vi "TH2829-20RunTest.vi"(0 "仪器通讯端口":refnum<visa-resource-name>, 6 "error in":errorcluster caption="错误输入（无错误）") -> (26 "error out":errorcluster caption="错误输出")   [LabVIEW 2018]
uses:
  Subvi/Global.vi
panel:
  out "数组 2":string[](array[string])
  out "数组":sgl[](array[numeric])
  out "子字符串":string
  out "read buffer":string
  out "Serial Settings:Number of Bytes at Serial Port":u32
  out "LED IrCompare Result":u8[][](array[numeric])
  out "LED IrResult":sgl[][](array[numeric]) format="%#_6f"
  out "总判断":u8
  out "Bls Result":sgl[][](array[numeric]) format="%#_6f"
  out "LED VfCompare Result":u8[][](array[numeric])
  out "LED VfResult":sgl[][](array[numeric]) format="%#_6f"
  out "PS Compare Result":u8[][](array[numeric])
  out "Polarity Result1":string[][](array[string])
  out "Rs Compare Result":u8[][](array[numeric])
  out "Z Compare Result":u8[][](array[numeric])
  out "Balance Compare Result":u8[][](array[numeric])
  out "LxQ Compare Result":u8[][](array[numeric])
  out "DCR Compare Result":u8[][](array[numeric])
  out "C Compare Result":u8[][](array[numeric])
  out "Lk Compare Result":u8[][](array[numeric])
  out "Lx Compare Result":u8[][](array[numeric])
  out "Turns Compare Result":u8[][](array[numeric])
  out "Polarity Result":u8[][](array[numeric])
  out "Zx Result":sgl[][](array[numeric]) format="%#_6f"
  out "ACR Result":sgl[][](array[numeric]) format="%#_6f"
  out "LxQ Result":sgl[][](array[numeric]) format="%#_6f"
  out "DCR Result":sgl[][](array[numeric]) format="%#_6f"
  out "Cx Result":sgl[][](array[numeric]) format="%#_6f"
  out "Lk Result":sgl[][](array[numeric]) format="%#_6f"
  out "Lx Result":sgl[][](array[numeric]) format="%#_6f"
  out "Turns Result":sgl[][](array[numeric]) format="%#_6f"
  out "Primary Sets":string
  out "head":string
  # "2304 0000 0000 0000 0000 0000 6041 E6C0 0B3D 0000 0000 F0A5 813C 0000 0000 0000 0000 0000 0000 0000 0000 0000 0000 0000 0000 0000 6041 3C18 E23C 0000 0000 CBA5 CD3B 0000 0000 0000 0000 0000 0000 0000 0000 0000 0000 0000 0000 0000 6041 D305 133D 0000 0000 5556 6A3C 0000 0000 0000 0000 0000 0000 0000 0000 0000 0000 0000 0000 0000 6041 A6B0 263D 0000 0000 2AAE 653C 0000 0000 0000 0000 0000 0000 0000 0000 0000 0000 0000 0000 0000 6041 072B 323D 0000 0000 A81B 993C 0000 0000 0000 0000 0000 0000 0000 0000 0000 0000 0000 0000 0000 6041 A94C 253D 0000 0000 D4A3 283C 0000 0000 0000 0000 0000 0000 0000 0000 0000 0000 0000 0000 0000 6041 849D 213D 0000 0000 39D1 7F3C 0000 0000 0000 0000 0000 0000 0000 0000 0000 0000 0000 0000 0000 6041 CA44 153D 0000 0000 3EC1 533C 0000 0000 0000 0000 0000 0000 0000 0000 0000 0000 0000 0000 0000 0000 0000 0000 0000 0000 0000 0000 0000 0000 0000 0000 0000 0000 0000 0000 0000 0000 0000 0000 0000 0000 0000 0000 0000 0000 0000 0000 0000 0000 0000 0000 0000 0000 0000 0000 0000 0000 0000 0000 0000 0000 0000 0000 0000 0000 0000 0000 0000 0000 0000 0000 0000 0000 0000 0000 0000 0000 0000 0000 0000 0000 0000 0000 0000 0000 0000 0000 0000 0000 0000 0000 0000 0000 0000 0000 0000 0000 0000 0000 0000 0000 0000 0000 0000 0000 0000 0000 0000 0000 0000 0000 0000 0000 0000 0000 0000 0000 0000 0000 0000 0000 0000 0000 0000 0000 0000 0000 0000 0000 0000 0000 0000 0000 0000 0000 0000 0000 0000 0000 0000 0000 0000 0000 0000 0000 0000 0000 0000 0000 0000 0000 0000 0000 0000 0000 0000 0000 0000 0000 0000 0000 0000 0000 0000 0000 0000 0000 0000 0000 0000 0000 0000 0000 0000 0000 0000 0000 0000 0000 0000 0000 0000 0000 0000 0000 0000 0000 0000 0000 0000 0000 0000 0000 0000 0000 0000 0000 0000 0000 0000 0000 0000 0000 0000 0000 0000 0000 0000 0000 0000 0000 0000 0000 0000 0000 0000 0000 0000 0000 0000 0000 0000 0000 0000 0000 0000 0000 0000 0000 0000 0000 0000 0000 0000 0000 0000 0000 0000 0000 0000 0000 0000 0000 0000 0000 0000 0000 0000 0000 0000 0000 0000 0000 0000 0000 0000 0000 0000 0000 0000 0000 0000 0000 0000 0000 0000 0000 0000 0000 0000 0000 0000 0000 0000 0000 0000 0000 0000 0000 0000 0000 0000 0000 0000 0000 0000 0000 0000 0000 0000 0000 0000 0000 0000 0000 0000 0000 0000 0000 0000 0000 0000 0000 0000 0000 0000 0000 0000 0000 0000 0000 0000 0000 0000 0000 0000 0000 0000 0000 0000 0000 0000 0000 0000 0000 0000 0000 0000 0000 0000 0000 0000 0000 0000 0000 0000 0000 0000 0000 0000 0000 0000 0000 0000 0000 0000 0000 0000 0000 0000 0000 0000 0000 0000 0000 0000 0000 0000 0000 0000 0000 0000 0000 0000 0000 0000 0000 0000 0000 0000 0000 0000 0000 0000 0000 0000 0000 0000 0000 0000 0000 0000 0000 0000 0000 0000 0000 0000 0000 0000 0000 0000 0000 0000 0000 0000 0000 0000 0000 0000 0000 0000 0000 0000 0000 0000 0000 0000 0000 0000 0000 0000 0000 0000 0000 0000 0000 0000 0000 0000 0000 0000 0000 0000 0000 0000 0000 0000 0000 0000 0000 0000 0000 0000 0000 0000 0000 0000 0000 0000 0000 0000 0000 0000 0000 0000 0000 0000 0000 0000 0000 0000 0000 0000 0000 0000 0000 0000 0000 0000 0000 0000 0000 0000 0000 0000 0000 0000 0000 0000 0000 0000 0000 0000 0000 0000 0000 0000 0000 0000 0000 0000 0000 0000 0000 0000 0000 0000 0000 0000 0000 0000 0000 0000 0000 0000 0000 0000 0000 0000 0000 0000 0000 0000 0000 0000 0000 0000 0000 0000 0000 0000 0000 0000 0000 0000 0000 0000 0000 0000 0000 0000 0000 0000 0000 0000 0000 0000 0000 0000 0000 0000 0000 0000 0000 0000 0000 0000 0000 0000 0000 0000 0000 0000 0000 0000 0000 0000 0000 0000 0000 0000 0000 0000 0000 0000 0000 0000 0000 0000 0000 0000 0000 0000 0000 0000 0000 0000 0000 0000 0000 0000 0000 0000 0000 0000 0000 0000 0000 0000 0000 0000 0000 0000 0000 0000 0000 0000 0000 0000 0000 0000 0000 0000 0000 0000 0000 0000 0000 0000 0000 0000 0000 0000 0000 0000 0000 0000 0000 0000 0000 0000 0000 0000 0000 0000 0000 0000 0000 0000 0000 0000 0000 0000 0000 0000 0000 0000 0000 0000 0000 0000 0000 0000 0000 0000 0000 0000 0000 0000 0000 0000 0000 0000 0000 0000 0000 0000 0000 0000 0000 0000 0000 0000 0000 0000 0000 0000 0000 F3AB 98BC 8E9F 1ABD 0000 0000 76B9 B1BD 0000 0000 0000 0000 0000 0000 0000 0000 0000 0000 0000 0000 75BB 8EBC 1715 01BD 0000 0000 76BC 77BD 0000 0000 0000 0000 0000 0000 0000 0000 0000 0000 0000 0000 A410 8FBC 4FD1 06BD 0000 0000 F5D1 79BD 0000 0000 0000 0000 0000 0000 0000 0000 0000 0000 0000 0000 DEEB A4BC 4F0C 15BD 0000 0000 485C 9CBD 0000 0000 0000 0000 0000 0000 0000 0000 0000 0000 0000 0000 06A7 86BC 0D51 1CBD 0000 0000 606A B1BD 0000 0000 0000 0000 0000 0000 0000 0000 0000 0000 0000 0000 209F A1BC 6393 02BD 0000 0000 2246 7BBD 0000 0000 0000 0000 0000 0000 0000 0000 0000 0000 0000 0000 AE0B 88BC 3FFC 07BD 0000 0000 BAB5 7FBD 0000 0000 0000 0000 0000 0000 0000 0000 0000 0000 0000 0000 459C 87BC C865 10BD 0000 0000 78DF 97BD 0000 0000 0000 0000 0000 0000 0000 0000 0000 0000 0000 0000 0000 0000 0000 0000 0000 0000 0000 0000 0000 0000 0000 0000 0000 0000 0000 0000 0000 0000 0000 0000 0000 0000 0000 0000 0000 0000 0000 0000 0000 0000 0000 0000 0000 0000 0000 0000 0000 0000 0000 0000 0000 0000 0000 0000 0000 0000 0000 0000 0000 0000 0000 0000 0000 0000 0000 0000 0000 0000 0000 0000 0000 0000 0000 0000 0000 0000 0000 0000 0000 0000 0000 0000 0000 0000 0000 0000 0000 0000 0000 0000 0000 0000 0000 0000 0000 0000 0000 0000 0000 0000 0000 0000 0000 0000 0000 0000 0000 0000 0000 0000 0000 0000 0000 0000 0000 0000 0000 0000 0000 0000 0000 0000 0000 0000 0000 0000 0000 0000 0000 0000 0000 0000 0000 0000 0000 0000 0000 0000 0000 0000 0000 0000 0000 0000 0000 0000 0000 0000 0000 0000 0000 0000 0000 0000 0000 0000 0000 0000 0000 0000 0000 0000 0000 0000 0000 0000 0000 0000 0000 0000 0000 0000 0000 0000 0000 0000 0000 0000 0000 0000 0000 0000 0000 0000 0000 0000 0000 0000 0000 0000 0000 0000 0000 0000 0000 0000 0000 0000 0000 0000 0000 0000 0000 0000 0000 0000 0000 0000 0000 0000 0000 0000 0000 0000 0000 0000 0000 0000 0000 0000 0000 0000 0000 0000 0000 0000 0000 0000 0000 0000 0000 0000 0000 0000 0000 0000 0000 0000 0000 0000 0000 0000 0000 0000 0000 0000 0000 0000 0000 0000 0000 0000 0000 0000 0000 0000 0000 0000 0000 0000 0000 0000 0000 0000 0000 0000 0000 0000 0000 0000 0000 0000 0000 0000 0000 0000 0000 0000 0000 0000 0000 0000 0000 0000 0000 0000 0000 0000 0000 0000 0000 0000 0000 0000 0000 0000 0000 0000 0000 0000 0000 0000 0000 0000 0000 0000 0000 0000 0000 0000 0000 0000 0000 0000 0000 0000 0000 0000 0000 0000 0000 0000 0000 0000 0000 0000 0000 0000 0000 0000 0000 0000 0000 0000 0000 0000 0000 0000 0000 0000 0000 0000 0000 0000 0000 0000 0000 0000 0000 0000 0000 0000 0000 0000 0000 0000 0000 0000 0000 0000 0000 0000 0000 0000 0000 0000 0000 0000 0000 0000 0000 0000 0000 0000 0000 0000 0000 0000 0000 0000 0000 0000 0000 0000 0000 0000 0000 0000 0000 0000 0000 0000 0000 0000 0000 0000 0000 0000 0000 0000 0000 0000 0000 0000 0000 0000 0000 0000 0000 0000 0000 0000 0000 0000 0000 0000 0000 0000 0000 0000 0000 0000 0000 0000 0000 0000 0000 0000 0000 0000 0000 0000 0000 0000 0000 0000 0000 0000 0000 0000 0000 0000 0000 0000 0000 0000 0000 0000 0000 0000 0000 0000 0000 0000 0000 0000 0000 0000 0000 0000 0000 0000 0000 0000 0000 0000 0000 0000 0000 0000 0000 0000 0000 0000 0000 0000 0000 0000 0000 0000 0000 0000 0000 0000 0000 0000 0000 0000 0000 0000 0000 0000 0000 0000 0000 0000 0000 0000 0000 0000 0000 0000 0000 0000 0000 0000 0000 0000 0000 0000 0000 0000 0000 0000 0000 0000 0000 0000 0000 0000 0000 0000 0000 0000 0000 0000 0000 0000 0000 0000 0000 0000 0000 0000 0000 0000 0000 0000 0000 0000 0000 0000 0000 0000 0000 0000 0000 0000 0000 0000 0000 0000 0000 0000 0000 0000 0000 0000 0000 0000 0000 0000 0000 0000 0000 0000 0000 0000 0000 0000 0000 0000 0000 0000 0000 0000 0000 0000 0000 0000 0000 0000 0000 0000 0000 0000 0000 0000 0000 0000 0000 0000 0000 0000 0000 0000 0000 0000 0000 0000 0000 0000 0000 0000 0000 0000 0000 0000 0000 0000 0000 0000 0000 0000 0000 0000 0000 0000 0000 0000 0000 0000 0000 0000 0000 0000 0000 0000 0000 0000 0000 0000 0000 0000 0000 0000 0000 0000 0000 0000 0000 0000 0000 0000 0000 0000 0000 0000 0000 0000 0000 0000 0000 0000 0000 0000 0000 0000 0000 0000 0000 0000 0000 0000 0000 0000 0000 0000 0000 0000 0000 0000 0000 0000 0000 0000 0000 0000 0000 0000 0000 0000 0000 0000 0000 0000 0000 0000 0000 0000 0000 0000 0000 0000 0000 0000 0000 0000 0000 0000 0000 0000 0000 0000 0000 0000 0000 0000 0000 0000 0000 0000 0000 0000 0000 0000 0000 0000 0000 0000 0000 0000 0000 0000 0000 0000 0000 0000 0000 0000 0000 0000 0000 0000 0000 0000 0000 0000 0000 0000 0000 0000 0000 0000 0000 0000 0000 0000 0000 0000 0000 0000 0000 0000 0000 0000 0000 0000 0000 0000 0000 0000 0000 0000 0000 0000 0000 0000 0000 0000 0000 0000 0000 0000 0000 0000 0000 0000 0000 0000 0000 0000 0000 0000 0000 0000 0000 0000 0000 0000 0000 0000 0000 0000 0000 0000 0000 0000 0000 0000 0000 0000 0000 0000 0000 0000 0000 0000 0000 0000 0000 0000 0000 0000 0000 0000 0000 0000 0000 0000 0000 0000 0000 0000 0000 0000 0000 0000 0000 0000 0000 0000 0000 0000 0000 0000 0000 0000 0000 0000 0000 0000 0000 0000 0000 0000 0000 0000 0000 0000 0000 0000 0000 0000 0000 0000 0000 0000 0000 0000 0000 0000 0000 0000 0000 0000 0000 0000 0000 0000 0000 0000 0000 0000 0000 0000 0000 0000 0000 0000 0000 0000 0000 0000 0000 0000 0000 0000 0000 0000 0000 0000 0000 0000 0000 0000 0000 0000 0000 0000 0000 0000 0000 0000 0000 0000 0000 0000 0000 0000 0000 0000 0000 0000 0000 0000 0000 0000 0000 0000 0000 0000 0000 0000 0000 0000 0000 0000 0000 0000 0000 0000 0000 0000 0000 0000 0000 0000 0000 0000 0000 0000 0000 0000 0000 0000 0000 0000 0000 0000 0000 0000 0000 0000 0000 0000 0000 0000 0000 0000 0000 0000 0000 0000 0000 0000 0000 0000 0000 0000 0000 0000 0000 0000 0000 0000 0000 0000 0000 0000 0000 0000 0000 0000 0000 0000 0000 0000 0000 0000 0000 0000 0000 0000 0000 0000 0000 0000 0000 0000 0000 0000 0000 0000 0000 0000 0000 0000 0000 0000 0000 0000 0000 0000 0000 0000 0000 0000 0000 0000 0000 0000 0000 0000 0000 0000 0000 0000 0000 0000 0000 0000 0000 0000 0000 0000 0000 0000 0000 0000 0000 0000 0000 0000 0000 0000 0000 0000 0000 0000 0000 0000 0000 0000 0000 0000 0000 0000 0000 0000 0000 0000 0000 0000 0000 0000 0000 0000 0000 0000 0000 0000 0000 0000 0000 0000 0000 0000 0000 0000 0000 0000 0000 0000 0000 0000 0000 0000 0000 0000 0000 0000 0000 0000 0000 0000 0000 0000 0000 0000 0000 0000 0000 0000 0000 0000 0000 0000 0000 0000 0000 0000 0000 0000 0000 0000 0000 0000 0000 0000 0000 0000 0000 0000 0000 0000 0000 0000 0000 0000 0000 0000 0000 0000 0000 0000 0000 0000 0000 0000 0000 0000 0000 0000 0000 0000 0000 0000 0000 0000 0000 0000 0000 0000 0000 0000 0000 0000 0000 0000 0000 0000 0000 0000 0000 0000 0000 0000 0000 0000 0000 0000 0000 0000 0000 0000 0000 0000 0000 0000 0000 0000 0000 0000 0000 0000 0000 0000 0000 0000 0000 0000 0000 0000 0000 0000 0000 0000 0000 0000 0000 0000 0000 0000 0000 0000 0000 0000 0000 0000 0000 0000 0000 0000 0000 0000 0000 0000 0000 0000 0000 0000 0000 0000 0000 0000 0000 0000 0000 0000 0000 0000 0000 0000 0000 0000 0000 0000 0000 0000 0000 0000 0000 0000 0000 0000 0000 0000 0000 0000 0000 0000 0000 0000 0000 0000 0000 0000 0000 0000 0000 0000 0000 0000 0000 0000 0000 0000 0000 0000 0000 0000 0000 0000 0000 0000 0000 0000 0000 0000 0000 0000 0000 0000 0000 0000 0000 0000 0000 0000 0000 0000 0000 0000 0000 0000 0000 0000 0000 0000 0000 0000 0000 0000 0000 0000 0000 0000 0000 0000 0000 0000 0000 0000 0000 0000 0000 0000 0000 0000 0000 0000 0000 0000 0000 0000 0000 0000 0000 0000 0000 0000 0000 0000 0000 0000 0000 0000 0000 0000 0000 0000 0000 0000 0000 0000 0000 0000 0000 0000 0000 0000 0000 0000 0000 0000 0000 0000 0000 0000 0000 0000 0000 0000 0000 0000 0000 0000 0000 0000 0000 0000 0000 0000 0000 0000 0000 0000 0000 0000 0000 0000 0000 0000 0000 0000 0000 0000 0000 0000 0000 0000 0000 0000 0000 0000 0000 0000 0000 0000 0000 0000 0000 0000 0000 0000 0000 0000 0000 0000 0000 0000 0000 0000 0000 0000 0000 0000 0000 0000 0000 0000 0000 0000 0000 0000 0000 0000 0000 0000 0000 0000 0000 0000 0000 0000 0000 0000 0000 0000 0000 0000 0000 0000 0000 0000 0000 0000 0000 0000 0000 0000 0000 0000 0000 0000 0000 0000 0000 0000 0000 0000 0000 0000 0000 0000 0000 0000 0000 0000 0000 0000 0000 0000 0000 0000 0000 0000 0000 0000 0000 0000 0000 0000 0000 0000 0000 0000 0000 0000 0000 0000 0000 0000 0000 0000 0000 0000 0000 0000 0000 0000 0000 0000 0000 0000 0000 0000 0000 0000 0000 0000 0000 0000 0000 0000 0000 0000 0000 0000 0000 0000 0000 0000 0000 0000 0000 0000 0000 0000 0000 0000 0000 0000 0000 0000 0000 0000 0000 0000 0000 0000 0000 0000 0000 0000 0000 0000 0000 0000 0000 0000 0000 0000 0000 0000 0000 0000 0000 0000 0000 0000 0000 0000 0000 0000 0000 0000 0000 0000 0000 0000 0000 0000 0000 0000 0000 0000 0000 0000 0000 0000 0000 0000 0000 0000 0000 0000 0000 0000 0000 0000 0000 0000 0000 0000 0000 0000 0000 0000 0000 0000 0000 0000 0000 0000 0000 0000 0000 0000 0000 0000 0000 0000 0000 0000 0000 0000 0000 0000 0000 0000 0000 0000 0000 0000 0000 0000 0000 0000 0000 0000 0000 0000 0000 0000 0000 0000 0000 0000 0000 0000 0000 0000 0000 0000 0000 0000 0000 0000 0000 0000 0000 0000 0000 0000 0000 0000 0000 0000 0000 0000 0000 0000 0000 0000 0000 0000 0000 0000 0000 0000 0000 0000 0000 0000 0000 0000 0000 0000 0000 0000 0000 0000 0000 0000 0000 0000 0000 0000 0000 0000 0000 0000 0000 0000 0000 0000 0000 0000 0000 0000 0000 0000 0000 0000 0000 0000 0000 0000 0000 0000 0000 0000 0000 0000 0000 0000 0000 0000 0000 0000 0000 0000 0000 0000 0000 0000 0000 0000 0000 0000 0000 0000 0000 0000 0000 0000 0000 0000 0000 0000 0000 0000 0000 0000 0000 0000 0000 0000 0000 0000 0000 0000 0000 0000 0000 0000 0000 0000 0000 0000 0000 0000 0000 0000 0000 0000 0000 0000 0000 0000 0000 0000 0000 0000 0000 0000 0000 0000 0000 0000 0000 0000 0000 0000 0000 0000 0000 0000 0000 0000 0000 0000 0000 0000 0000 0000 0000 0000 0000 0000 0000 0000 0000 0000 0000 0000 0000 0000 0000 0000 0000 0000 0000 0000 0000 0000 0000 0000 0000 0000 0000 0000 0000 0000 0000 0000 0000 0000 0000 0000 0000 0000 0000 0000 0000 0000 0000 0000 0000 0000 0000 0000 0000 0000 0000 0000 0000 0000 0000 0000 0000 0000 0000 0000 0000 0000 0000 0000 0000 0000 0000 0000 0000 0000 0000 0000 0000 0000 0000 0000 0000 0000 0000 0000 0000 0000 0000 0000 0000 0000 0000 0000 0000 0000 0000 0000 0000 0000 0000 0000 0000 0000 0000 0000 0000 0000 0000 0000 0000 0000 0000 0000 0000 0000 0000 0000 0000 0000 0000 0000 0000 0000 0000 0000 0000 0000 0000 0000 0000 0000 0000 0000 0000 0000 0000 0000 0000 0000 0000 0000 0000 0000 0000 0000 0000 0000 0000 0000 0000 0000 0000 0000 0000 0000 0000 0000 0000 0000 0000 0000 0000 0000 0000 0000 0000 0000 0000 0000 0000 0000 0000 0000 0000 0000 0000 0000 0000 0000 0000 0000 0000 0000 0000 0000 0000 0000 0000 0000 0000 0000 0000 0000 0000 0000 0000 0000 0000 0000 0000 0000 0000 0000 0000 0000 0000 0000 0000 0000 0000 0000 0000 0000 0000 0000 0000 0000 0000 0000 0000 0000 0000 0000 0000 0000 0000 0000 0000 0000 0000 0000 0000 0000 0000 0000 0000 0000 0000 0000 0000 0000 0000 0000 0000 0000 0000 0000 0000 0000 0000 0000 0000 0000 0000 0000 0000 0000 0000 0000 0000 0000 0000 0000 0000 0000 0000 0000 0000 0000 0000 0000 0000 0000 0000 0000 0000 0000 0000 0000 0000 0000 0000 0000 0000 0000 0000 0000 0000 0000 0000 0000 0000 0000 0000 0000 0000 0000 0000 0000 0000 0000 0000 0000 0000 0000 0000 0000 0000 0000 0000 0000 0000 0000 0000 0000 0000 0000 0000 0000 0000 0000 0000 0000 0000 0000 0000 0000 0000 0000 0000 0000 0000 0000 0000 0000 0000 0000 0000 0000 0000 0000 0000 0000 0000 0000 0000 0000 0000 0000 0000 0000 0000 0000 0000 0000 0000 0000 0000 0000 0000 0000 0000 0000 0000 0000 0000 0000 0000 0000 0000 0000 0000 0000 0000 0000 0000 0000 0000 0000 0000 0000 0000 0000 0000 0000 0000 0000 0000 0000 0000 0000 0000 0000 0000 0000 0000 0000 0000 0000 0000 0000 0000 0000 0000 0000 0000 0000 0000 0000 0000 0000 0000 0000 0000 0000 0000 0000 0000 0000 0000 0000 0000 0000 0000 0000 0000 0000 0000 0000 0000 0000 0000 0000 0000 0000 0000 0000 0000 0000 0000 0000 0000 0000 0000 0000 0000 0000 0000 0000 0000 0000 0000 0000 0000 0000 0000 0000 0000 0000 C79E 2E47 B30A 2148 6078 544C 3046 5A47 0000 0000 0000 0000 0000 0000 0000 0000 0000 0000 0000 0000 959E 2E47 2DF0 1048 6078 544C F446 5A47 0000 0000 0000 0000 0000 0000 0000 0000 0000 0000 0000 0000 FC9E 2E47 130B 2148 9CE8 3B4C 1547 5A47 0000 0000 0000 0000 0000 0000 0000 0000 0000 0000 0000 0000 7C9F 2E47 C3F0 1048 436B 744C 869F 2E47 0000 0000 0000 0000 0000 0000 0000 0000 0000 0000 0000 0000 ED90 2E47 9AE4 1048 7748 744C 0435 5A47 0000 0000 0000 0000 0000 0000 0000 0000 0000 0000 0000 0000 0991 2E47 82E4 1048 A648 744C 2435 5A47 0000 0000 0000 0000 0000 0000 0000 0000 0000 0000 0000 0000 A190 2E47 6FE4 1048 A648 744C DC90 2E47 0000 0000 0000 0000 0000 0000 0000 0000 0000 0000 0000 0000 8890 2E47 941D 3548 4A48 744C 2135 5A47 0000 0000 0000 0000 0000 0000 0000 0000 0000 0000 0000 0000 0000 0000 0000 0000 0000 0000 0000 0000 0000 0000 0000 0000 0000 0000 0000 0000 0000 0000 0000 0000 0000 0000 0000 0000 0000 0000 0000 0000 0000 0000 0000 0000 0000 0000 0000 0000 0000 0000 0000 0000 0000 0000 0000 0000 0000 0000 0000 0000 0000 0000 0000 0000 0000 0000 0000 0000 0000 0000 0000 0000 0000 0000 0000 0000 0000 0000 0000 0000 0000 0000 0000 0000 0000 0000 0000 0000 0000 0000 0000 0000 0000 0000 0000 0000 0000 0000 0000 0000 0000 0000 0000 0000 0000 0000 0000 0000 0000 0000 0000 0000 0000 0000 0000 0000 0000 0000 0000 0000 0000 0000 0000 0000 0000 0000 0000 0000 0000 0000 0000 0000 0000 0000 0000 0000 0000 0000 0000 0000 0000 0000 0000 0000 0000 0000 0000 0000 0000 0000 0000 0000 0000 0000 0000 0000 0000 0000 0000 0000 0000 0000 0000 0000 0000 0000 0000 0000 0000 0000 0000 0000 0000 0000 0000 0000 0000 0000 0000 0000 0000 0000 0000 0000 0000 0000 0000 0000 0000 0000 0000 0000 0000 0000 0000 0000 0000 0000 0000 0000 0000 0000 0000 0000 0000 0000 0000 0000 0000 0000 0000 0000 0000 0000 0000 0000 0000 0000 0000 0000 0000 0000 0000 0000 0000 0000 0000 0000 0000 0000 0000 0000 0000 0000 0000 0000 0000 0000 0000 0000 0000 0000 0000 0000 0000 0000 0000 0000 0000 0000 0000 0000 0000 0000 0000 0000 0000 0000 0000 0000 0000 0000 0000 0000 0000 0000 0000 0000 0000 0000 0000 0000 0000 0000 0000 0000 0000 0000 0000 0000 0000 0000 0000 0000 0000 0000 0000 0000 0000 0000 0000 0000 0000 0000 0000 0000 0000 0000 0000 0000 0000 0000 0000 0000 0000 0000 0000 0000 0000 0000 0000 0000 0000 0000 0000 0000 0000 0000 0000 0000 0000 0000 0000 0000 0000 0000 0000 0000 0000 0000 0000 0000 0000 0000 0000 0000 0000 0000 0000 0000 0000 0000 0000 0000 0000 0000 0000 0000 0000 0000 0000 0000 0000 0000 0000 0000 0000 0000 0000 0000 0000 0000 0000 0000 0000 0000 0000 0000 0000 0000 0000 0000 0000 0000 0000 0000 0000 0000 0000 0000 0000 0000 0000 0000 0000 0000 0000 0000 0000 0000 0000 0000 0000 0000 0000 0000 0000 0000 0000 0000 0000 0000 0000 0000 0000 0000 0000 0000 0000 0000 0000 0000 0000 0000 0000 0000 0000 0000 0000 0000 0000 0000 0000 0000 0000 0000 0000 0000 0000 0000 0000 0000 0000 0000 0000 0000 0000 0000 0000 0000 0000 0000 0000 0000 0000 0000 0000 0000 0000 0000 0000 0000 0000 0000 0000 0000 0000 0000 0000 0000 0000 0000 0000 0000 0000 0000 0000 0000 0000 0000 0000 0000 0000 0000 0000 0000 0000 0000 0000 0000 0000 0000 0000 0000 0000 0000 0000 0000 0000 0000 0000 0000 0000 0000 0000 0000 0000 0000 0000 0000 0000 0000 0000 0000 0000 0000 0000 0000 0000 0000 0000 0000 0000 0000 0000 0000 0000 0000 0000 0000 0000 0000 0000 0000 0000 0000 0000 0000 0000 0000 0000 0000 0000 0000 0000 0000 0000 0000 0000 0000 0000 0000 0000 0000 0000 0000 0000 0000 0000 0000 0000 0000 0000 0000 0000 0000 0000 0000 0000 0000 0000 0000 0000 0000 0000 0000 0000 0000 0000 0000 0000 0000 0000 0000 0000 0000 0000 0000 0000 0000 0000 0000 0000 0000 0000 0000 0000 0000 0000 0000 0000 0000 0000 0000 0000 0000 0000 0000 0000 0000 0000 0000 0000 0000 0000 0000 0000 0000 0000 0000 0000 0000 0000 0000 0000 0000 0000 0000 0000 0000 0000 0000 0000 0000 0000 0000 0000 0000 0000 0000 0000 0000 0000 0000 0000 0000 0000 0000 0000 0000 0000 0000 0000 0000 0000 0000 0000 0000 0000 0000 0000 0000 3B8C 48C3 E13C 88C2 0000 0000 E8AF C241 0000 0000 0000 0000 0000 0000 0000 0000 0000 0000 0000 0000 C165 2DC2 C9E0 C4C2 0000 0000 7FA3 1B42 0000 0000 0000 0000 0000 0000 0000 0000 0000 0000 0000 0000 832E 59C2 11B7 CB42 0000 0000 80F2 C541 0000 0000 0000 0000 0000 0000 0000 0000 0000 0000 0000 0000 CE1C F542 118C 09C3 0000 0000 D11B 0342 0000 0000 0000 0000 0000 0000 0000 0000 0000 0000 0000 0000 D29F 36C2 66F9 F8C2 0000 0000 1C9A A941 0000 0000 0000 0000 0000 0000 0000 0000 0000 0000 0000 0000 3882 DA41 CB53 EEC2 0000 0000 013E 1042 0000 0000 0000 0000 0000 0000 0000 0000 0000 0000 0000 0000 4C13 2A43 CF61 C542 0000 0000 318A BE41 0000 0000 0000 0000 0000 0000 0000 0000 0000 0000 0000 0000 1D63 0FC2 B6B2 B2C2 0000 0000 7420 0042 0000 0000 0000 0000 0000 0000 0000 0000 0000 0000 0000 0000 0000 0000 0000 0000 0000 0000 0000 0000 0000 0000 0000 0000 0000 0000 0000 0000 0000 0000 0000 0000 0000 0000 0000 0000 0000 0000 0000 0000 0000 0000 0000 0000 0000 0000 0000 0000 0000 0000 0000 0000 0000 0000 0000 0000 0000 0000 0000 0000 0000 0000 0000 0000 0000 0000 0000 0000 0000 0000 0000 0000 0000 0000 0000 0000 0000 0000 0000 0000 0000 0000 0000 0000 0000 0000 0000 0000 0000 0000 0000 0000 0000 0000 0000 0000 0000 0000 0000 0000 0000 0000 0000 0000 0000 0000 0000 0000 0000 0000 0000 0000 0000 0000 0000 0000 0000 0000 0000 0000 0000 0000 0000 0000 0000 0000 0000 0000 0000 0000 0000 0000 0000 0000 0000 0000 0000 0000 0000 0000 0000 0000 0000 0000 0000 0000 0000 0000 0000 0000 0000 0000 0000 0000 0000 0000 0000 0000 0000 0000 0000 0000 0000 0000 0000 0000 0000 0000 0000 0000 0000 0000 0000 0000 0000 0000 0000 0000 0000 0000 0000 0000 0000 0000 0000 0000 0000 0000 0000 0000 0000 0000 0000 0000 0000 0000 0000 0000 0000 0000 0000 0000 0000 0000 0000 0000 0000 0000 0000 0000 0000 0000 0000 0000 0000 0000 0000 0000 0000 0000 0000 0000 0000 0000 0000 0000 0000 0000 0000 0000 0000 0000 0000 0000 0000 0000 0000 0000 0000 0000 0000 0000 0000 0000 0000 0000 0000 0000 0000 0000 0000 0000 0000 0000 0000 0000 0000 0000 0000 0000 0000 0000 0000 0000 0000 0000 0000 0000 0000 0000 0000 0000 0000 0000 0000 0000 0000 0000 0000 0000 0000 0000 0000 0000 0000 0000 0000 0000 0000 0000 0000 0000 0000 0000 0000 0000 0000 0000 0000 0000 0000 0000 0000 0000 0000 0000 0000 0000 0000 0000 0000 0000 0000 0000 0000 0000 0000 0000 0000 0000 0000 0000 0000 0000 0000 0000 0000 0000 0000 0000 0000 0000 0000 0000 0000 0000 0000 0000 0000 0000 0000 0000 0000 0000 0000 0000 0000 0000 0000 0000 0000 0000 0000 0000 0000 0000 0000 0000 0000 0000 0000 0000 0000 0000 0000 0000 0000 0000 0000 0000 0000 0000 0000 0000 0000 0000 0000 0000 0000 0000 0000 0000 0000 0000 0000 0000 0000 0000 0000 0000 0000 0000 0000 0000 0000 0000 0000 0000 0000 0000 0000 0000 0000 0000 0000 0000 0000 0000 0000 0000 0000 0000 0000 0000 0000 0000 0000 0000 0000 0000 0000 0000 0000 0000 0000 0000 0000 0000 0000 0000 0000 0000 0000 0000 0000 0000 0000 0000 0000 0000 0000 0000 0000 0000 0000 0000 0000 0000 0000 0000 0000 0000 0000 0000 0000 0000 0000 0000 0000 0000 0000 0000 0000 0000 0000 0000 0000 0000 0000 0000 0000 0000 0000 0000 0000 0000 0000 0000 0000 0000 0000 0000 0000 0000 0000 0000 0000 0000 0000 0000 0000 0000 0000 0000 0000 0000 0000 0000 0000 0000 0000 0000 0000 0000 0000 0000 0000 0000 0000 0000 0000 0000 0000 0000 0000 0000 0000 0000 0000 0000 0000 0000 0000 0000 0000 0000 0000 0000 0000 0000 0000 0000 0000 0000 0000 0000 0000 0000 0000 0000 0000 0000 0000 0000 0000 0000 0000 0000 0000 0000 0000 0000 0000 0000 0000 0000 0000 0000 0000 0000 0000 0000 0000 0000 0000 0000 0000 0000 0000 0000 0000 0000 0000 0000 0000 0000 0000 0000 0000 0000 0000 0000 0000 0000 0000 0000 0000 0000 0000 0000 0000 0000 0000 0000 0000 0000 0000 0000 0000 0000 0000 0000 0000 0000 0000 0000 0000 0000 0000 0000 0000 0000 0000 0000 0000 0000 0000 0000 0000 0000 0000 0000 0000 0000 0000 0000 0000 0000 0000 0000 0000 0000 0000 0000 0000 0000 0000 0000 0000 0000 0000 0000 0000 0000 0000 0000 0000 0000 0000 0000 0000 0000 0000 0000 0000 0000 0000 0000 0000 0000 0000 0000 0000 0000 0000 0000 0000 0000 0000 0000 0000 0000 0000 0000 0000 0000 0000 0000 0000 0000 0000 0000 0000 0000 0000 0000 0000 0000 0000 0000 0000 0000 0000 0000 0000 0000 0000 0000 0000 0000 0000 0000 0000 0000 0000 0000 0000 0000 0000 0000 0000 0000 0000 0000 0000 0000 0000 0000 0000 0000 0000 0000 0000 0000 0000 0000 0000 0000 0000 0000 0000 0000 0000 0000 0000 0000 0000 0000 0000 0000 0000 0000 0000 0000 0000 0000 0000 0000 0000 0000 0000 0000 0000 0000 0000 0000 0000 0000 0000 0000 0000 0000 0000 0000 0000 0000 0000 0000 0000 0000 0000 0000 0000 0000 0000 0000 0000 0000 0000 0000 0000 0000 0000 0000 0000 0000 0000 0000 0000 0000 0000 0000 0000 0000 0000 0000 0000 0000 0000 0000 0000 0000 0000 0000 0000 0000 0000 0000 0000 0000 0000 0000 0000 0000 0000 0000 0000 0000 0000 0000 0000 0000 0000 0000 0000 0000 0000 0000 0000 0000 0000 0000 0000 0000 0000 0000 0000 0000 0000 0000 0000 0000 0000 0000 0000 0000 0000 0000 0000 0000 0000 0000 0000 0000 0000 0000 0000 0000 0000 0000 0000 0000 0000 0000 0000 0000 0000 0000 0000 0000 0000 0000 0000 0000 0000 0000 0000 0000 0000 0000 0000 0000 0000 0000 0000 0000 0000 0000 0000 0000 0000 0000 0000 0000 0000 0000 0000 0000 0000 0000 0000 0000 0000 0000 0000 0000 0000 0000 0000 0000 0000 0000 0000 0000 0000 0000 0000 0000 0000 0000 0000 0000 0000 0000 0000 0000 0000 0000 0000 0000 0000 0000 0000 0000 0000 0000 0000 0000 0000 0000 0000 0000 0000 0000 0000 0000 0000 0000 0000 0000 0000 0000 0000 0000 0000 0000 0000 0000 0000 0000 0000 0000 0000 0000 0000 0000 0000 0000 0000 0000 0000 0000 0000 0000 0000 0000 0000 0000 0000 0000 0000 0000 0000 0000 0000 0000 0000 0000 0000 0000 0000 0000 0000 0000 0000 0000 0000 0000 0000 0000 0000 0000 0000 0000 0000 0000 0000 0000 0000 0000 0000 0000 0000 0000 0000 0000 0000 0000 0000 0000 0000 0000 0000 0000 0000 0000 0000 0000 0000 0000 0000 0000 0000 0000 0000 0000 0000 0000 0000 0000 0000 0000 0000 0000 0000 0000 0000 0000 0000 0000 0000 0000 0000 0000 0000 0000 0000 0000 0000 0000 0000 0000 0000 0000 0000 0000 0000 0000 0000 0000 0000 0000 0000 0000 0000 0000 0000 0000 0000 0000 0000 0000 0000 0000 0000 0000 0000 0000 0000 0000 0000 0000 0000 0000 0000 0000 0000 0000 0000 0000 0000 0000 0000 0000 0000 0000 0000 0000 0000 0000 0000 0000 0000 0000 0000 0000 0000 0000 0000 0000 0000 0000 0000 0000 0000 0000 0000 0000 0000 0000 0000 0000 0000 0000 0000 0000 0000 0000 0000 0000 0000 0000 0000 0000 0000 0000 0000 0000 0000 0000 0000 0000 0000 0000 0000 0000 0000 0000 0000 0000 0000 0000 0000 0000 0000 0000 0000 0000 0000 0000 0000 0000 0000 0000 0000 0000 0000 0000 0000 0000 0000 0000 0000 0000 0000 0000 0000 0000 0000 0000 0000 0000 0000 0000 0000 0000 0000 0000 0000 0000 0000 0000 0000 0000 0000 0000 0000 0000 0000 0000 0000 0000 0000 0000 0000 0000 0000 0000 0000 0000 0000 0000 0000 0000 0000 0000 0000 0000 0000 0000 0000 0000 0000 0000 0000 0000 0000 0000 0000 0000 0000 0000 0000 0000 0000 0000 0000 0000 0000 0000 0000 0000 0000 0000 0000 0000 0000 0000 0000 0000 0000 0000 0000 0000 0000 0000 0000 0000 0000 0000 0000 0000 0000 0000 0000 0000 0000 0000 0000 0000 0000 0000 0000 0000 0000 0000 0000 0000 0000 0000 0000 0000 0000 0000 0000 0000 0000 0000 0000 0000 0000 0000 0000 0000 0000 0000 0000 0000 0000 0000 0000 0000 0000 0000 0000 0000 0000 0000 0000 0000 0000 0000 0000 0000 0000 0000 0000 0000 0000 0000 0000 0000 0000 0000 0000 0000 0000 0000 0000 0000 0000 0000 0000 0000 0000 0000 0000 0000 0000 0000 0000 0000 0000 0000 0000 0000 0000 0000 0000 0000 0000 0000 0000 0000 0000 0000 0000 0000 0000 0000 0000 0000 0000 0000 0000 0000 0000 0000 0000 0000 0000 0000 0000 0000 0000 0000 0000 0000 0000 0000 0000 0000 0000 0000 0000 0000 0000 0000 0000 0000 0000 0000 0000 0000 0000 0000 0000 0000 0000 0000 0000 0000 0000 0000 0000 0000 0000 0000 0000 0000 0000 0000 0000 0000 0000 0000 0000 0000 0000 0000 0000 0000 0000 0000 0000 0000 0000 0000 0000 0000 0000 0000 0000 0000 0000 0000 0000 0000 0000 0000 0000 0000 0000 0000 0000 0000 0000 0000 0000 0000 0000 0000 0000 0000 0000 0000 0000 0000 0000 0000 0000 0000 0000 0000 0000 0000 0000 0000 0000 0000 0000 0000 0000 0000 0000 0000 0000 0000 0000 0000 0000 0000 0000 0000 0000 0000 0000 0000 0000 0000 0000 0000 0000 0000 0000 0000 0000 0000 0000 0000 0000 0000 0000 0000 0000 0000 0000 0000 0000 0000 0000 0000 0000 0000 0000 0000 0000 0000 0000 0000 0000 0000 0000 0000 0000 0000 0000 0000 0000 0000 0000 0000 0000 0000 0000 0000 0000 0000 0000 0000 0000 0000 0000 0000 0000 0000 0000 0000 0000 0000 0000 0000 0000 0000 0000 0000 0000 0000 0000 0000 0000 0000 0000 0000 0000 0000 0000 0000 0000 0000 0000 0000 0000 0000 0000 0000 0000 0000 0000 0000 0000 0000 0000 0000 0000 0000 0000 0000 0000 0000 0000 0000 0000 0000 0000 0000 0000 0000 0000 0000 0000 0000 0000 0000 0000 0000 0000 0000 0000 0000 0000 0000 0000 0000 0000 0000 0000 0000 0000 0000 0000 0000 0000 0000 0000 0000 0000 0000 0000 0000 0000 0000 0000 0000 0000 0000 0000 0000 0000 0000 0000 0000 0000 0000 0000 0000 0000 0000 0000 0000 0000 0000 0000 0000 0000 0000 0000 0000 0000 0000 0000 0000 0000 0000 0000 0000 0000 0000 0000 0000 0000 0000 0000 0000 0000 0000 0000 0000 0000 0000 0000 0000 0000 0000 0000 0000 0000 0000 0000 0000 0000 0000 0000 0000 0000 0000 0000 0000 0000 0000 0000 0000 0000 0000 0000 0000 0000 0000 0000 0000 0000 0000 0000 0000 0000 0000 0000 0000 0000 0000 0000 0000 0000 0000 0000 0000 0000 0000 0000 0000 0000 0000 0000 0000 0000 0000 0000 0000 0000 0000 0000 0000 0000 0000 0000 0000 0000 0000 0000 0000 0000 0000 0000 0000 0000 0000 0000 0000 0000 0000 0000 0000 0000 0000 0000 0000 0000 0000 0000 0000 0000 0000 0000 0000 0000 0000 0000 0000 0000 0000 0000 0000 0000 0000 0000 0000 0000 0000 0000 0000 0000 0000 0000 0000 0000 0000 0000 0000 0000 0000 0000 0000 0000 0000 0000 0000 0000 0000 0000 0000 0000 0000 0000 0000 0000 0000 0000 0000 0000 0000 0000 0000 0000 0000 0000 0000 0000 0000 0000 0000 0000 0000 0000 0000 0000 0000 0000 0000 0000 0000 0000 0000 0000 0000 0000 0000 0000 0000 0000 0000 0000 0000 0000 0000 0000 0000 0000 0000 0000 0000 0000 0000 0000 0000 0000 0000 0000 0000 0000 0000 0000 0000 0000 0000 0000 0000 0000 0000 0000 0000 0000 0000 0000 0000 0000 0000 0000 0000 0000 0000 0000 0000 0000 0000 0000 0000 0000 0000 0000 0000 0000 0000 0000 0000 0000 0000 0000 0000 0000 0000 0000 0000 0000 0000 0000 0000 0000 0000 0000 0000 0000 0000 0000 0000 0000 0000 0000 0000 0000 0000 0000 0000 0000 0000 0000 0000 0000 0000 0000 0000 0000 0000 0000 0000 0000 0000 0000 0000 0000 0000 0000 0000 0000 0000 0000 0000 0000 0000 0000 0000 0000 0000 0000 0000 0000 0000 0000 0000 0000 0000 0000 0000 0000 0000 0000 0000 0000 0000 0000 0000 0000 0000 0000 0000 0000 0000 0000 0000 0000 0000 0000 0000 0000 0000 0000 0000 0000 0000 0000 0000 0000 0000 0000 0000 0000 0000 0000 0000 0000 0000 0000 0000 0000 0000 0000 0000 0000 0000 0000 0000 0000 0000 0000 0000 0000 0000 0000 0000 0000 0000 0000 0000 0000 0000 0000 0000 0000 0000 0000 0000 0000 0000 0000 0000 0000 0000 0000 0000 0000 0000 0000 0000 0000 0000 0000 0000 0000 0000 0000 0000 0000 0000 0000 0000 0000 0000 0000 0000 0000 0000 0000 0000 0000 0000 0000 0000 0000 0000 0000 0000 0000 0000 0000 0000 0000 0000 0000 0000 0000 0000 0000 0000 0000 0000 0000 0000 0000 0000 0000 0000 0000 0000 0000 0000 0000 0000 0000 0000 0000 0000 0000 0000 0000 0000 0000 0000 0000 0000 0000 0000 0000 0000 0000 0000 0000 0000 0000 0000 0000 0000 0000 0000 0000 0000 0000 0000 0000 0000 0000 0000 0000 0000 0000 0000 0000 0000 0000 0000 0000 0000 0000 0000 0000 0000 0000 0000 0000 0000 0000 0000 0000 0000 0000 0000 0000 0000 0000 0000 0000 0000 0000 0000 0000 0000 0000 0000 0000 0000 0000 0000 0000 0000 0000 0000 0000 0000 0000 0000 0000 0000 0000 0000 0000 0000 0000 0000 0000 0000 0000 0000 0000 0000 0000 0000 0000 0000 0000 0000 0000 0000 0000 0000 0000 0000 0000 0000 0000 0000 0000 0000 0000 0000 0000 0000 0000 0000 0000 0000 0000 0000 0000 0000 0000 0000 0000 0000 0000 0000 0000 0000 0000 0000 2B2D 202D 2020 2020 2020 2B2D 202D 2020 2020 2020 2B2D 202D 2020 2020 2020 2B2D 202D 2020 2020 2020 2B2D 202D 2020 2020 2020 2B2D 202D 2020 2020 2020 2B2D 202D 2020 2020 2020 2B2D 202D 2020 2020 2020 2020 2020 2020 2020 2020 2020 2020 2020 2020 2020 2020 2020 2020 2020 2020 2020 2020 2020 2020 2020 2020 2020 2020 2020 2020 2020 2020 2020 2020 2020 2020 2020 2020 2020 2020 2020 2020 2020 2020 2020 2020 2020 2020 2020 2020 2020 2020 2020 2020 2020 2020 2020 2020 2020 2020 2020 2020 2020 2020 2020 2020 2020 2020 2020 2020 2020 2020 2020 2020 2020 2020 2020 2020 2020 2020 2020 2020 2020 2020 2020 2020 2020 2020 2020 2020 2020 2020 2020 2020 2020 2020 2020 2020 2020 2020 2020 2020 2020 2020 2020 2020 2020 2020 2020 2020 2020 2020 2020 2020 2020 2020 2020 2020 2020 2020 2020 2020 2020 2020 2020 2020 2020 2020 2020 2020 2020 2020 2020 2020 2020 2020 2020 2020 2020 2020 2020 2020 2020 2020 2020 2020 2020 2020 2020 2020 2020 2020 2020 2020 2020 2020 2020 2020 2020 2020 2020 2020 2020 2020 2020 0002 0002 0000 0000 0000 0002 0002 0000 0000 0000 0002 0002 0000 0000 0000 0002 0002 0000 0000 0000 0002 0002 0000 0000 0000 0002 0002 0000 0000 0000 0002 0002 0000 0000 0000 0002 0002 0000 0000 0000 0000 0000 0000 0000 0000 0000 0000 0000 0000 0000 0000 0000 0000 0000 0000 0000 0000 0000 0000 0000 0000 0000 0000 0000 0000 0000 0000 0000 0000 0000 0000 0000 0000 0000 0000 0000 0000 0000 0000 0000 0000 0000 0000 0000 0000 0000 0000 0000 0000 0000 0000 0000 0000 0000 0000 0000 0000 0000 0000 0000 0000 0000 0000 0000 0000 0000 0000 0000 0000 0000 0000 0000 0000 0000 0000 0000 0000 0000 0000 0000 0000 0000 0000 0000 0000 0000 0000 0000 0000 0000 0000 0000 0000 0000 0000 0000 0000 0000 0000 0000 0000 0000 0000 0000 0000 0000 0000 0000 0000 0000 0000 0000 0000 0000 0000 0000 0000 0000 0000 0000 0000 0000 0000 0000 0000 0000 0000 0000 0000 0000 0000 0000 0000 0000 0000 0000 0000 0000 0000 0000 0000 0000 0000 0000 0000 0000 0000 0000 0000 0000 0000 0000 0000 0000 0000 0000 0000 0000 0000 0000 0202 0002 0000 0000 0000 0202 0002 0000 0000 0000 0202 0002 0000 0000 0000 0202 0002 0000 0000 0000 0202 0002 0000 0000 0000 0202 0002 0000 0000 0000 0202 0002 0000 0000 0000 0202 0002 0000 0000 0000 0000 0000 0000 0000 0000 0000 0000 0000 0000 0000 0000 0000 0000 0000 0000 0000 0000 0000 0000 0000 0000 0000 0000 0000 0000 0000 0000 0000 0000 0000 0000 0000 0000 0000 0000 0000 0000 0000 0000 0000 0000 0000 0000 0000 0000 0000 0000 0000 0000 0000 0000 0000 0000 0000 0000 0000 0000 0000 0000 0000 0000 0000 0000 0000 0000 0000 0000 0000 0000 0000 0000 0000 0000 0000 0000 0000 0000 0000 0000 0000 0000 0000 0000 0000 0000 0000 0000 0000 0000 0000 0000 0000 0000 0000 0000 0000 0000 0000 0000 0000 0000 0000 0000 0000 0000 0000 0000 0000 0000 0000 0000 0000 0000 0000 0000 0000 0000 0000 0000 0000 0000 0000 0000 0000 0000 0000 0000 0000 0000 0000 0000 0000 0000 0000 0000 0000 0000 0000 0000 0000 0000 0000 0000 0000 0000 0000 0000 0000 0000 0000 0000 0000 0000 0000 0000 0000 0000 0000 0000 0000 0000 0000 0000 0000 0000 0000 0000 0000 0000 0000 0000 0000 0000 0000 0000 0000 0000 0000 0000 0000 0000 0000 0000 0000 0000 0000 0000 0000 0000 0000 0000 0000 0000 0000 0000 0000 0000 0000 0000 0000 0000 0000 0000 0000 0000 0000 0000 0000 0000 0000 0000 0000 0000 0000 0000 0000 0000 0000 0000 0000 0000 0000 0000 0000 0000 0000 0000 0000 0000 0000 0000 0000 0000 0000 0000 0000 0000 0000 0000 0000 0000 0000 0000 0000 0000 0000 0000 0000 0000 0000 0000 0000 0000 0000 0000 0000 0000 0000 0000 0000 0000 0000 0000 0000 0000 0000 0000 0000 0000 0000 0000 0000 0000 0000 0000 0000 0000 0000 0000 0000 0000 0000 0000 0000 0000 0000 0000 0000 0000 0000 0000 0000 0000 0000 0000 0000 0000 0000 0000 0000 0000 0000 0000 0000 0000 0000 0000 0000 0000 0000 0000 0000 0000 0000 0000 0000 0000 0000 0000 0000 0000 0000 0000 0000 0000 0000 0000 0000 0000 0000 0000 0000 0000 0000 0000 0000 0000 0000 0000 0000 0000 0000 0000 0000 0000 0000 0000 0000 0000 0000 0000 0000 0000 0000 0000 0000 0000 0000 0000 0000 0000 0000 0000 0000 0000 0000 0000 0000 0000 0000 0000 0000 0000 0000 0000 0000 0000 0000 0000 0000 0000 0000 0000 0000 0000 0000 0000 0000 0000 0000 0000 0000 0000 0000 0000 0000 0000 0000 0000 0000 0000 0000 0000 0000 0000 0000 0000 0000 0000 0000 0000 0000 0000 0000 0000 0000 0000 0000 0000 0000 0000 0000 0000 0000 0000 0000 0000 0000 0000 0000 0000 0000 0000 0000 0000 0000 0000 0000 0000 0000 0000 0000 0000 0000 0000 0000 0000 0000 0000 0000 0000 0000 0000 0000 0000 0000 0000 0000 0000 0000 0000 0000 0000 0000 0000 0000 0000 0000 0000 0000 0000 0000 0000 0000 0000 0000 0000 0000 0000 0000 0000 0000 0000 0000 0000 0000 0000 0000 0000 0000 0000 0000 0000 0000 0000 0000 0000 0000 0000 0000 0000 0000 0000 0000 0000 0000 0000 0000 0000 0000 0000 0000 0000 0000 0000 0000 0000 0000 0000 0000 0000 0000 0000 0000 0000 0000 0000 0000 0000 0000 0000 0000 0000 0000 0000 0000 0000 0000 0000 0000 0000 0000 0000 0000 0000 0000 0000 0000 0000 0000 0000 0000 0000 0000 0000 0000 0000 0000 0000 0000 0303 0303 0000 0000 0000 0303 0303 0000 0000 0000 0303 0303 0000 0000 0000 0303 0303 0000 0000 0000 0303 0303 0000 0000 0000 0303 0303 0000 0000 0000 0303 0303 0000 0000 0000 0303 0303 0000 0000 0000 0000 0000 0000 0000 0000 0000 0000 0000 0000 0000 0000 0000 0000 0000 0000 0000 0000 0000 0000 0000 0000 0000 0000 0000 0000 0000 0000 0000 0000 0000 0000 0000 0000 0000 0000 0000 0000 0000 0000 0000 0000 0000 0000 0000 0000 0000 0000 0000 0000 0000 0000 0000 0000 0000 0000 0000 0000 0000 0000 0000 0000 0000 0000 0000 0000 0000 0000 0000 0000 0000 0000 0000 0000 0000 0000 0000 0000 0000 0000 0000 0000 0000 0000 0000 0000 0000 0000 0000 0000 0000 0000 0000 0000 0000 0000 0000 0000 0000 0000 0000 0000 0000 0000 0000 0000 0000 0000 0000 0000 0000 0000 0000 0000 0000 0000 0000 0000 0000 0000 0000 0000 0000 0000 0000 0000 0000 0000 0000 0000 0000 0000 0000 0000 0000 0000 0000 0000 0000 0000 0000 0000 0000 0000 0000 0000 0000 0000 0000 0000 0000 0000 0000 0000 0000 0000 0000 0000 0000 0000 0000 0000 0000 0000 0000 0000 0000 0000 0000 0000 0000 0000 0000 0000 0000 0000 0000 0000 0000 0000 0000 0000 0000 0000 0000 0000 0000 0000 0000 0000 0000 0000 0000 0000 0000 0000 0000 0000 0000 0000 0000 0000 0000 0000 0000 0000 0000 0000 0000 0000 0000 0000 0000 0000 0000 0000 0000 0000 0000 0000 0000 0000 0000 0000 0000 0000 0000 0000 0000 0000 0000 0000 0000 0000 0000 0000 0000 0000 0000 0000 0000 0000 0000 0000 0000 0000 0000 0000 0000 0000 0000 0000 0000 0000 0000 0000 0000 0000 0000 0000 0000 0000 0000 0000 0000 0000 0000 0000 0000 0000 0000 0000 0000 0000 0000 0000 0000 0000 0000 0000 0000 0000 0000 0000 0000 0000 0000 0000 0000 0000 0000 0000 0000 0000 0000 0000 0000 0000 0000 0000 0000 0000 0000 0000 0000 0000 0000 0000 0000 0000 0000 0000 0000 0000 0000 0000 0000 0000 0000 0000 0000 0000 0000 0000 0000 0000 0000 0000 0000 0000 0000 0000 0000 0000 0000 0000 0000 0000 0000 0000 0000 0000 0000 0000 0000 0000 0000 0000 0000 0000 0000 0000 0000 0000 0000 0000 0000 0000 0000 0000 0000 0000 0000 0000 0000 0000 0000 0000 0000 0000 0000 0000 0000 0000 0000 0000 0000 0000 0000 0000 0000 0000 0000 0000 0000 0000 0000 0000 0000 0000 0000 0000 0000 0000 0000 0000 0000 0000 0000 0000 0000 0000 0000 0000 0000 0000 0000 0000 0000 0000 0000 0000 0000 0000 0000 0000 0000 0000 0000 0000 0000 0000 0000 0000 0000 0000 0000 0000 0000 0000 0000 0000 0000 0000 0000 0000 0000 0000 0000 0000 0000 0000 0000 0000 0000 0000 0000 0000 0000 0000 0000 0000 0000 0000 0000 0000 0000 0000 0000 0000 0000 0000 0000 0000 0000 0000 0000 0000 0000 0000 0000 0000 0000 0000 0000 0000 0000 0000 0000 0000 0000 0000 0000 0000 0000 0000 0000 0000 0000 0000 0000 0000 0000 0000 0000 0000 0000 0000 0000 0000 0000 0000 0000 0000 0000 0000 0000 0000 0000 0000 0000 0000 0000 0000 0000 0000 0000 0000 0000 0000 0000 0000 0000 0000 0000 0000 0000 0000 0000 0000 0000 0000 0000 0000 0000 0000 0000 0000 0000 0000 0000 0000 0000 0000 0000 0000 0000 0000 0000 0000 0000 0000 0000 0000 0000 0000 0000 0000 0000 0000 0000 0000 0000 0000 0000 0000 0000 0000 0000 0000 0000 0000 0000 0000 0000 0000 0000 0000 0000 0000 0000 0000 0000 0000 0000 0000 0000 0000 0000 0000 0000 0000 0000 0000 0000 0000 0000 0000 0000 0000 0000 0000 0000 0000 0000 0000 0000 0000 0000 0000 0000 0000 0000 0000 0000 0000 0000 0000 0000 0000 0000 0000 0000 0000 0000 0000 0000 0000 0000 0000 0000 0000 0000 0000 0000 0000 0000 0000 0000 0000 0000 0000 0000 0000 0000 0000 0000 0000 0000 0000 0000 0000 0000 0000 0000 0000 0000 0000 0000 0000 0000 0000 0000 0000 0000 0000 0000 0000 0000 0000 0000 0000 0000 0000 0000 0000 0000 0000 0000 0000 0000 0000 0000 0000 0000 0000 0000 0000 0000 0000 0000 0000 0000 0000 0000 0000 0000 0000 0000 0000 0000 0000 0000 0000 0000 0000 0000 0000 0000 0000 0000 0000 0000 0000 0000 0000 0000 0000 0000 0000 0000 0000 0000 0000 0000 0000 0000 0000 0000 0000 0000 0000 0000 0000 0000 0000 0000 0000 0000 0000 0000 0000 0000 0000 0000 0000 0000 0000 0000 0000 0000 0000 0000 0000 0000 0000 0000 0000 0000 0000 0000 0000 0000 0000 0000 0000 0000 0000 0000 0000 0000 0000 0000 0000 0000 0000 0000 0000 0000 0000 0000 0000 0000 0000 0000 0000 0000 0000 0000 0000 0000 0000 0000 0000 0000 0000 0000 0000 0000 0000 0000 0000 0000 0000 0000 0000 0000 0000 0000 0000 0000 0000 0000 0000 0000 0000 0000 0000 0000 0000 0000 0000 0000 0000 0000 0000 0000 0000 0000 0000 0000 0000 0000 0000 0000 0000 0000 0000 0000 0000 0000 0000 0000 0000 0000 0000 0000 0000 0000 0000 0000 0000 0000 0000 0000 0000 0000 0000 0000 0000 0000 0000 0000 0000 0000 0000 0000 0000 0000 0000 0000 0000 0000 0000 0000 0000 0000 0000 0000 0000 0000 0000 0000 0000 0000 0000 0000 0000 0000 0000 0000 0000 0000 0000 0000 0000 0000 0000 0000 0000 0000 0000 0000 0000 0000 0000 0000 0000 0000 0000 0000 0000 0000 0000 0000 0000 0000 0000 0000 0000 0000 0000 0000 0000 0000 0000 0000 0000 0000 0000 0000 0000 0000 0000 0000 0000 0000 0000 0000 0000 0000 0000 0000 0000 0000 0000 0000 0000 0000 0000 0000 0000 0000 0000 0000 0000 0000 0000 0000 0000 0000 0000 0000 0000 0000 0000 0000 0000 0000 0000 0000 0000 0000 0000 0000 0000 0000 0000 0000 0000 0000 0000 0000 0000 0000 0000 0000 0000 0000 0000 0000 0000 0000 0000 0000 0000 0000 0000 0000 0000 0000 0000 0000 0000 0000 0000 0000 0000 0000 0000 0000 0000 0000 0000 0000 0000 0000 0000 0000 0000 0000 0000 0000 0000 0000 0000 0000 0000 0000 0000 0000 0000 0000 0000 0000 0000 0000 0000 0000 0000 0000 0000 0000 0000 0000 0000 0000 0000 0000 0000 0000 0000 0000 0000 0000 0000 0000 0000 0000 0000 0000 0000 0000 0000 0000 0000 0000 0000 0000 0000 0000 0000 0000 0000 0000 0000 0000 0000 0000 0000 0000 0000 0000 0000 0000 0000 0000 0000 0000 0000 0000 0000 0000 0000 0000 0000 0000 0000 0000 0000 0000 0000 0000 0000 0000 0000 0000 0000 0000 0000 0000 0000 0000 0000 0000 0000 0000 0000 0000 0000 0000 0000 0000 0000 0000 0000 0000 0000 0000 0000 0000 0000 0000 0000 0000 0000 0000 0000 0000 0000 0000 0000 0000 0000 0000 0000 0000 0000 0000 0000 0000 0000 0000 0000 0000 0000 0000 0000 0000 0000 0000 0400 0000 0000 0000 0000 0000 0000 0000 0000 0000 0000 0000 0000 0000 0000 0000 0000 0000 0000 0000 0000 0000 0000 0000 0000 0000 0000 0000 0000 0000 0000 0000 0000 0000 0000 0000 0000 0000 0000 0000 0000 0000 0000 0000 0000 0000 0000 0000 0000 0000 0000 0000 0000 0000 0000 0000 0000 0000 0000 0000 0000 0000 0000 0000 0000 0000 0000 0000 0000 0000 0000 0000 0000 0000 0000 0000 0000 0000 0000 0000 0000 0000 0000 0000 0000 0000 0000 0000 0000 0000 0000 0000 0000 0000 0000 0000 0000 0000 0000 0000 0000 0000 0000 0000 0000 0000 0000 0000 0000 0000 0000 0000 0000 0000 0000 0000 0000 0000 0000 0000 0000 0000 0000 0000 0000 0000 0000 0000 0000 0000 0000 0000 0000 0000 0000 0000 0000 0000 0000 0000 0000 0000 0000 0000 0000 0000 0000 0000 0000 0000 0000 0000 0000 0000 0000 0000 0000 0000 0000 0000 0000 0000 0000 0000 0000 0000 0000 0000 0000 0000 0000 0000 0000 0000 0000 0000 0000 0000 0000 0000 0000 0000 0000 0000 0000 0000 0000 0000 0000 0000 0000 0000 0000 0000 0000 0000 0000 0000 0000 0000 0000 0000 0000 0000 0000 0000 0000 0000 0000 0000 0000 0000 0000 0000 0000 0000 0000 0000 0000 0000 0000 0000 0000 0000 0000 0000 0000 0000 0000 0000 0000 0000 0000 0000 0000 0000 0000 0000 0000 0000 0000 0000 0000 0000 0000 0000 0000 0000 0000 0000 0000 0000 0000 0000 0000 0000 0000 0000 0000 0000 0000 0000 0000 0000 0000 0000 0000 0000 0000 0000 0000 0000 0000 0000 0000 0000 0000 0000 0000 0000 0000 0000 0000 0000 0000 0000 0000 0000 0000 0000 0000 0000 0000 0000 0000 0000 0000 0000 0000 0000 0000 0000 0000 0000 0000 0000 0000 0000 0000 0000 0000 0000 0000 0000 0000 0000 0000 0000 0000 0000 0000 0000 0000 0000 0000 0000 0000 0000 0000 0000 0000 0000 0000 0000 0000 0000 0000 0000 0000 0000 0000 0000 0000 0000 0000 0000 0000 0000 0000 0000 0000 0000 0000 0000 0000 0000 0000 0000 0000 0000 0000 0000 0000 0000 0000 0000 0000 0000 0000 0000 0000 0000 0000 0000 0000 0000 0000 0000 0000 0000 0000 0000 0000 0000 0000 0000 0000 0000 0000 0000 0000 0000 0000 0000 0000 0000 0000 0000 0000 0000 0000 0000 0000 0000 0000 0000 0000 0000 0000 0000 0000 0000 0000 0000 0000 0000 0000 0000 0000 0000 0000 0000 0000 0000 0000 0000 0000 0000 0000 0000 0000 0000 0000 0000 0000 0000 0000 0000 0000 0000 0000 0000 0000 0000 0000 0000 0000 0000 0000 0000 0000 0000 0000 0000 0000 0000 0000 0000 0000 0000 0000 0000 0000 0000 0000 0000 0000 0000 0000 0000 0000 0000 0000 0000 0000 0000 0000 0000 0000 0000 0000 0000 0000 0000 0000 0000 0000 0000 0000 0000 0000 0000 0000 0000 0000 0000 0000 0000 0000 0000 0000 0000 0000 0000 0000 0000 0000 0000 0000 0000 0000 0000 0000 0000 0000 0000 0000 0000 0000 0000 0000 0000 0000 0000 0000 0000 0000 0000 0000 0000 0000 0000 0000 0000 0000 0000 0000 0000 0000 0000 0000 0000 0000 0000 0000 0000 0000 0000 0000 0000 0000 0000 0000 0000 0000 0000 0000 0000 0000 0000 0000 0000 0000 0000 0000 0000 0000 0000 0000 0000 0000 0000 0000 0000 0000 0000 0000 0000 0000 0000 0000 0000 0000 0000 0000 0000 0000 0000 0000 0000 0000 0000 0000 0000 0000 0000 0000 0000 0000 0000 0000 0000 0000 0000 0000 0000 0000 0000 0000 0000 0000 0000 0000 0000 0000 0000 0000 0000 0000 0000 0000 0000 0000 0000 0000 0000 0000 0000 0000 0000 0000 0000 0000 0000 0000 0000 0000 0000 0000 0000 0000 0000 0000 0000 0000 0000 0000 0000 0000 0000 0000 0000 0000 0000 0000 0000 0000 0000 0000 0000 0000 0000 0000 0000 0000 0000 0000 0000 0000 0000 0000 0000 0000 0000 0000 0000 0000 0000 0000 0000 0000 0000 0000 0000 0000 0000 0000 0000 0000 0000 0000 0000 0000 0000 0000 0000 0000 0000 0000 0000 0000 0000 0000 0000 0000 0000 0000 0000 0000 0000 0000 0000 0000 0000 0000 0000 0000 0000 0000 0000 0000 0000 0000 0000 0000 0000 0000 0000 0000 0000 0000 0000 0000 0000 0000 0000 0000 0000 0000 0000 0000 0000 0000 0000 0000 0000 0000 0000 0000 0000 0000 0000 0000 0000 0000 0000 0000 0000 0000 0000 0000 0000 0000 0000 0000 0000 0000 0000 0000 0000 0000 0000 0000 0000 0000 0000 0000 0000 0000 0000 0000 0000 0000 0000 0000 0000 0000 0000 0000 0000 0000 0000 0000 0000 0000 0000 0000 0000 0000 0000 00"
  # "0000 6041 4CE2 0B3D 0000 0000 56E5 813C"
  # "4160 0000 3D0B E24C 0000 0000 3C81 E556"
  # "0.0341515"
  # "0.0158564"
  # "14"
  # "0"
  # "0.0275935"
  # "0.0063041"
  # "14"
  # "0"
  # "0.03596"
  # "0.0143324"
  # "0"
  # "14"
  # "0.0406281"
  # "0.0140537"
  # "14"
  # "0"
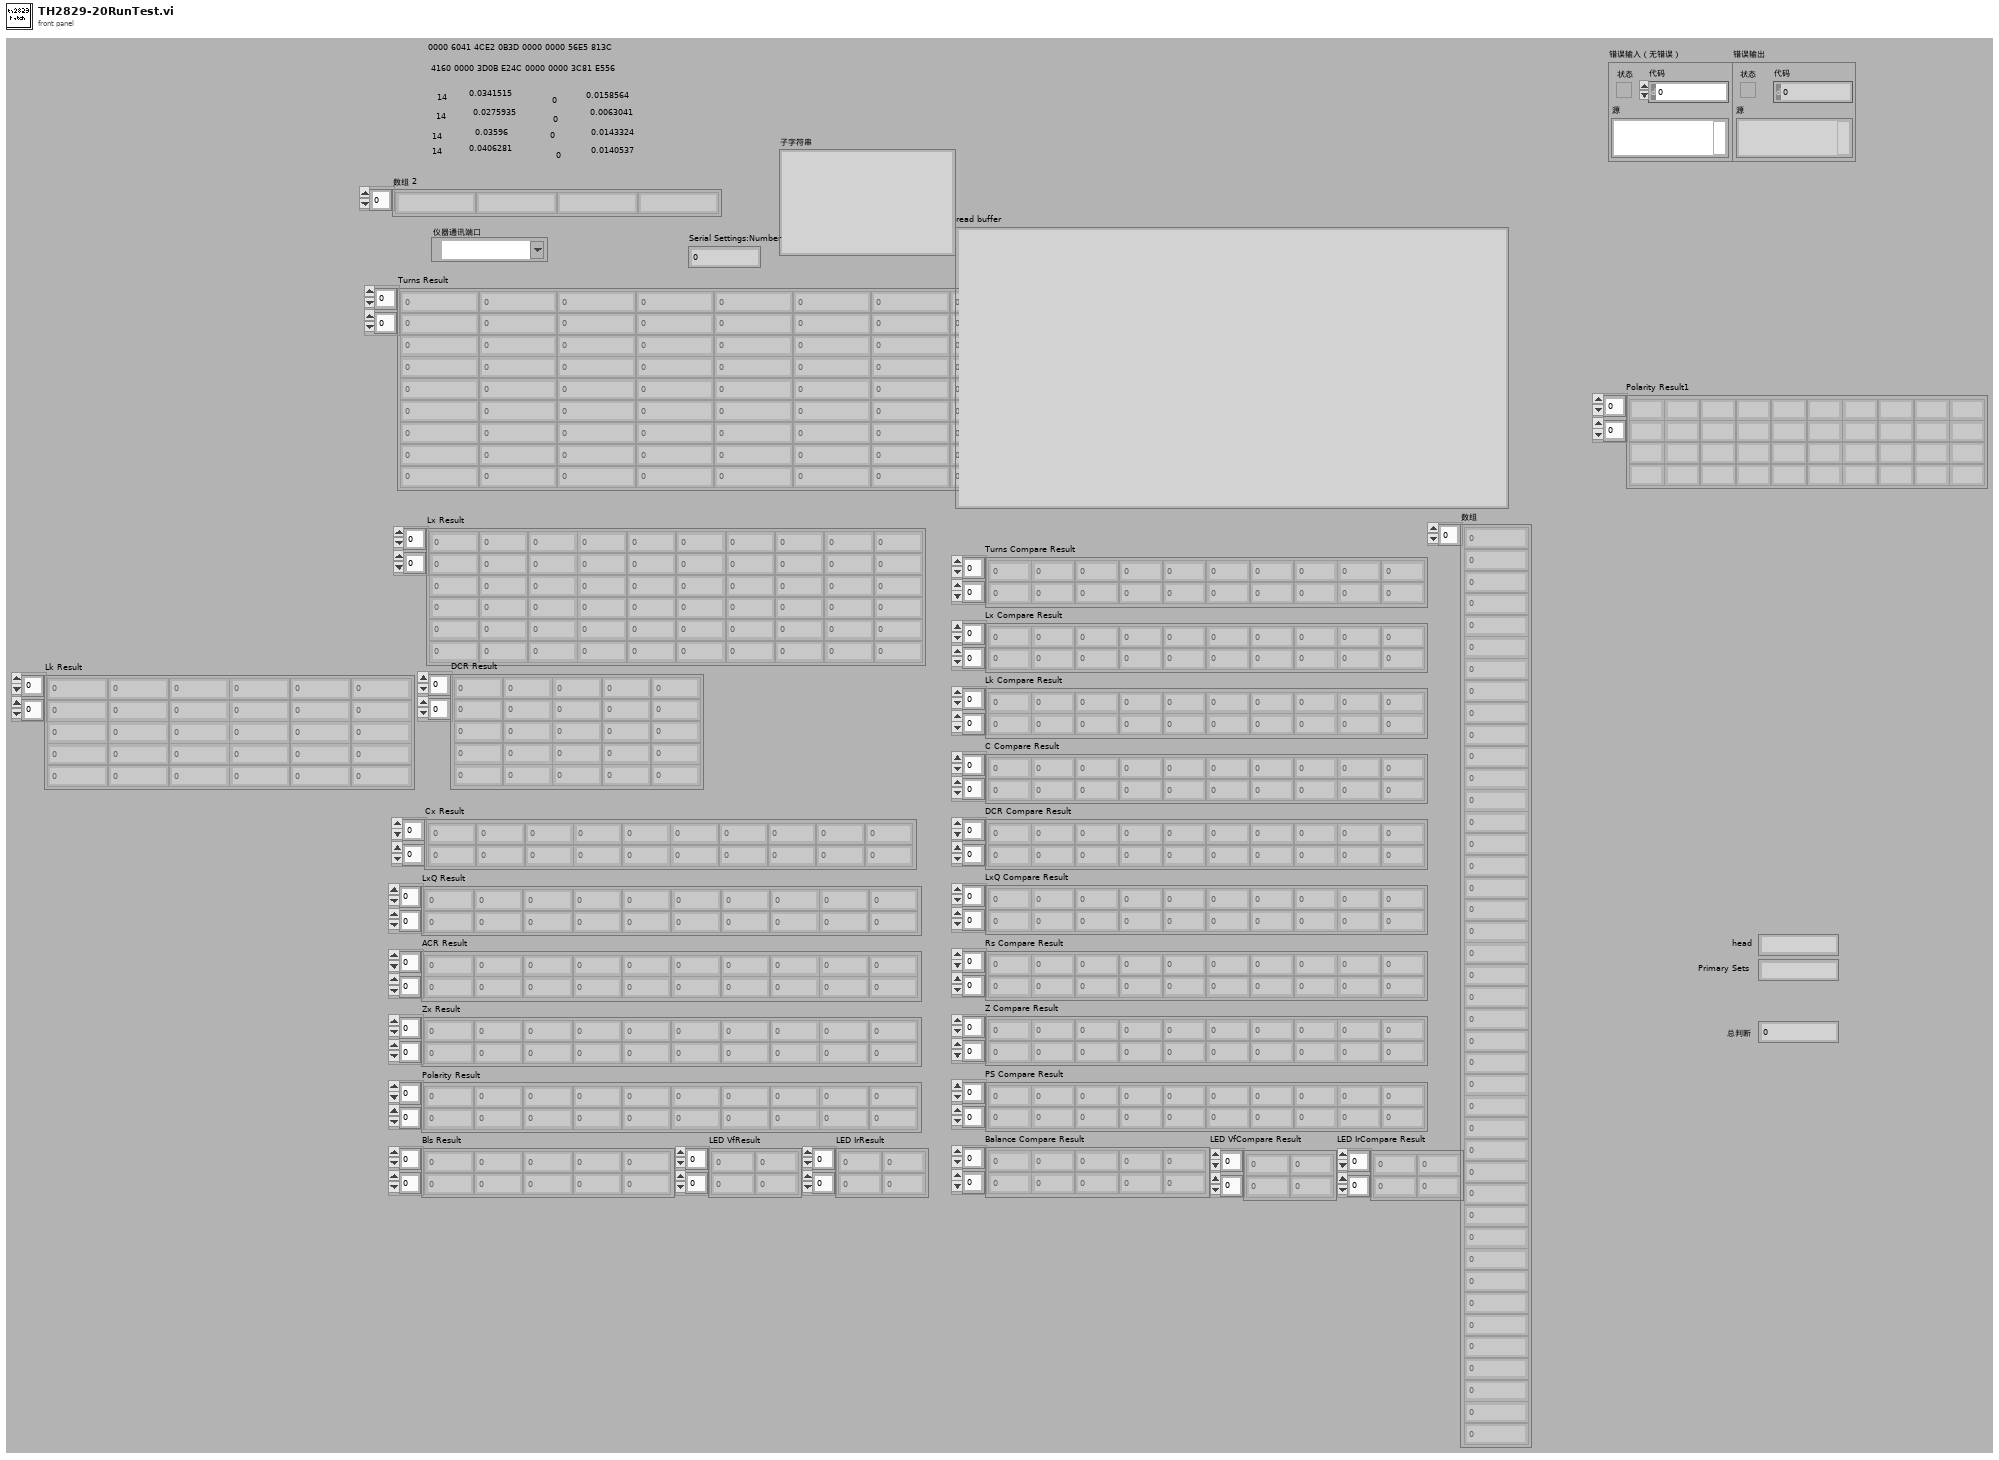
[diagram p1: front panel]
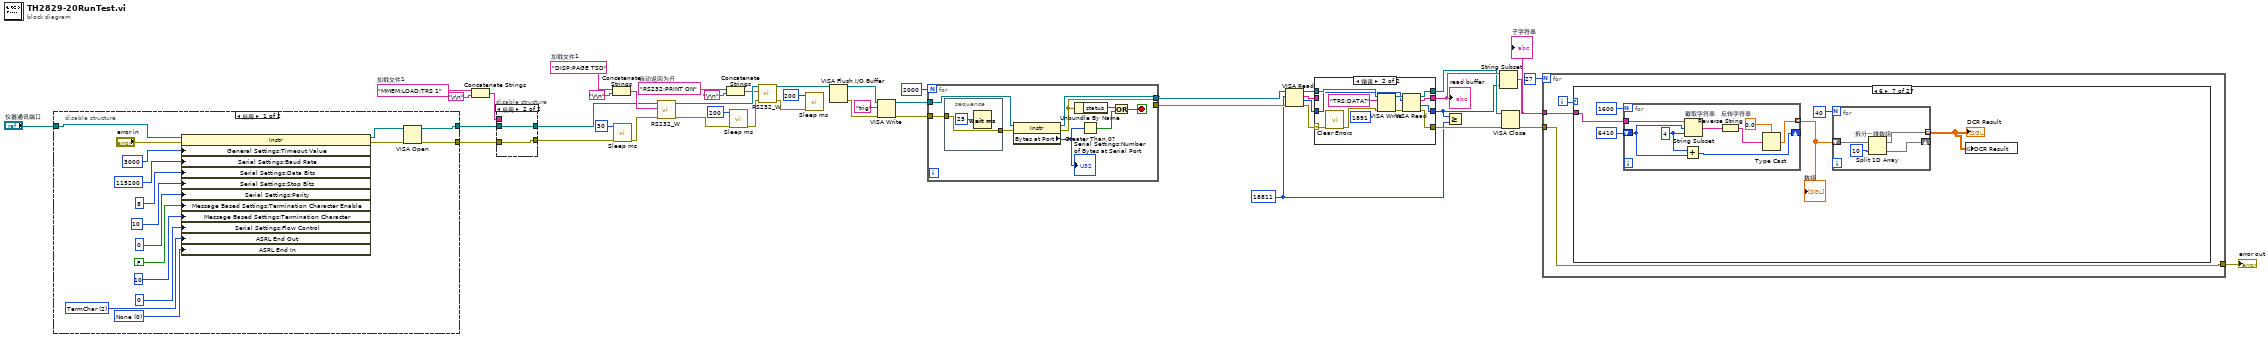
[diagram p0: block diagram]
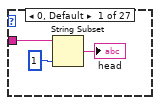
[diagram p2: hidden frame]
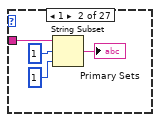
[diagram p3: hidden frame]
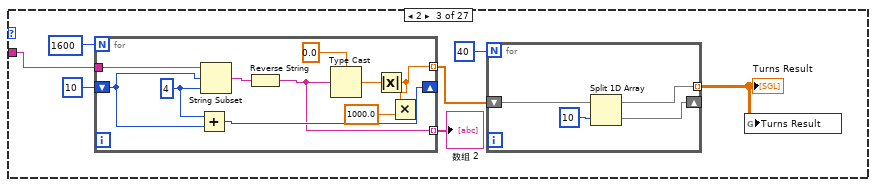
[diagram p4: hidden frame]
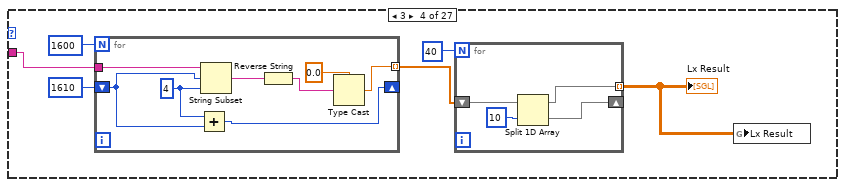
[diagram p5: hidden frame]
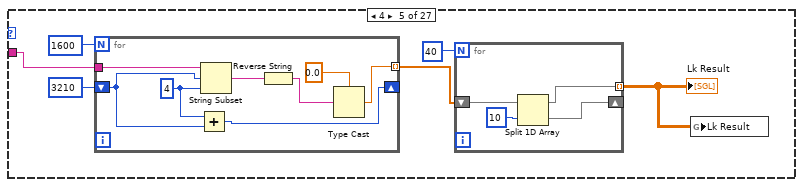
[diagram p6: hidden frame]
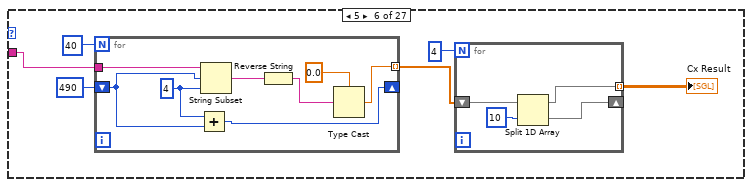
[diagram p7: hidden frame]
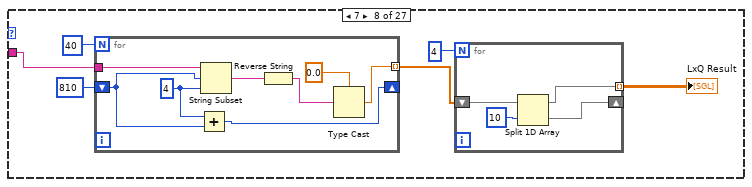
[diagram p8: hidden frame]
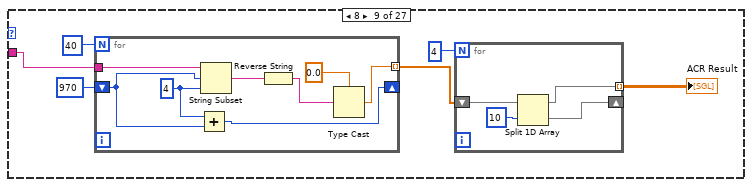
[diagram p9: hidden frame]
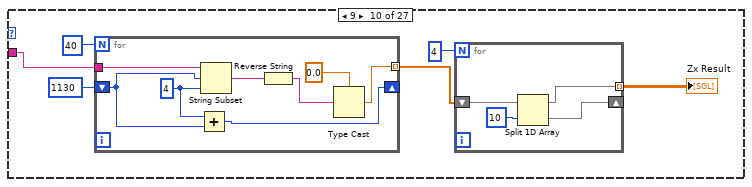
[diagram p10: hidden frame]
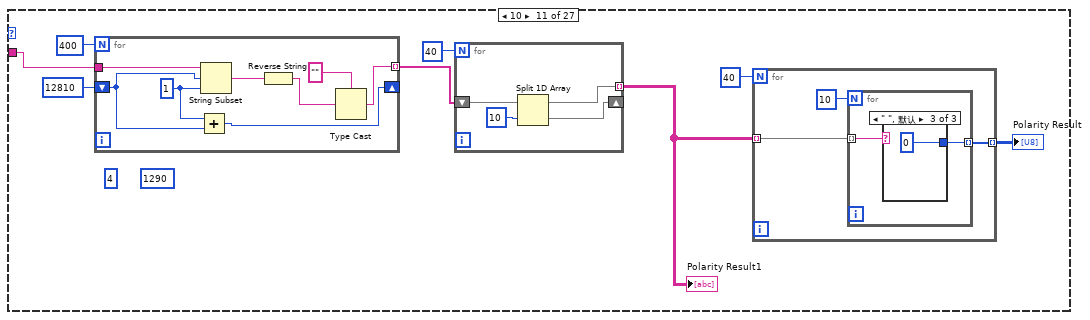
[diagram p11: hidden frame]
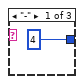
[diagram p12: hidden frame]
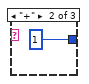
[diagram p13: hidden frame]
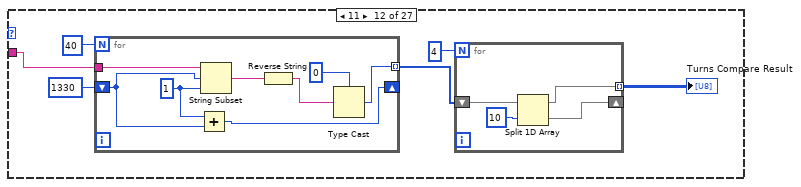
[diagram p14: hidden frame]
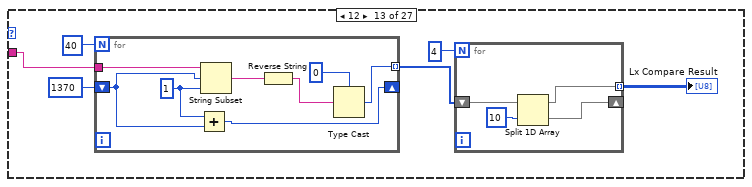
[diagram p15: hidden frame]
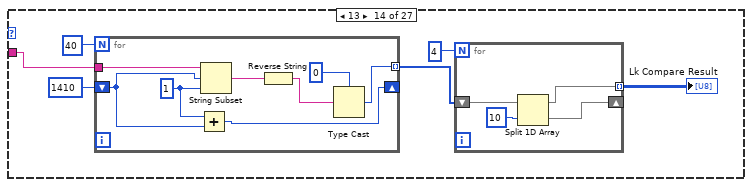
[diagram p16: hidden frame]
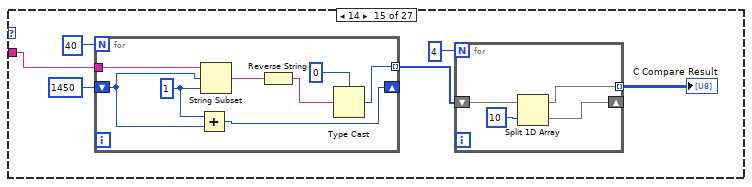
[diagram p17: hidden frame]
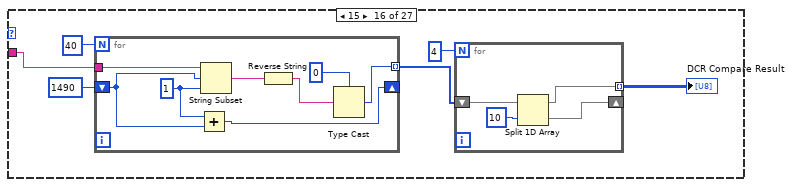
[diagram p18: hidden frame]
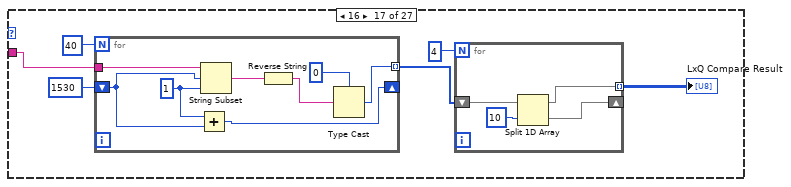
[diagram p19: hidden frame]
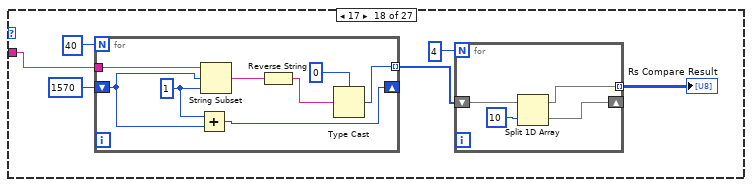
[diagram p20: hidden frame]
diagram:
  w11 = "MMEM:LOAD:TRS 1"  # 加载文件1
  w13 = "RS232:PRINT ON"  # 自动返回为开
  w14 = "DISP:PAGE TSD"  # 加载文件1
  w32 = u32 18811 ("字节总数")
  n1 = disable-structure shown="启用" {
    disable-tunnel: [w60 w61] -> w9
    disable-tunnel: [w59 _] -> w8
    disable-tunnel: "仪器通讯端口" -> [w56 w61]
    frame Enabled {
      w49 = u16 0 items=["None", "Last Bit", "TermChar"] ("Serial Settings:End Mode for Reads")
      w51 = u16 2 items=["None", "Last Bit", "TermChar", "Break"] ("Serial Settings:End Mode for Writes")
      n2 = property class="Instr"(reference=w56, error in="error in", "General Settings:Timeout Value"=u32 3000, "Serial Settings:Baud Rate"=u32 115200, "Serial Settings:Data Bits"=u16 8, "Serial Settings:Stop Bits"=u16 10, "Serial Settings:Parity"=u16 0, "Message Based Settings:Termination Character Enable"=FALSE ("TermChar En"), "Message Based Settings:Termination Character"=u8 10, "Serial Settings:Flow Control"=u16 0, "ASRL End Out"=w51, "ASRL End In"=w49) -> (reference out=w57:refnum<visa-resource-name>, error out=w58:errorcluster)
      n3 = VISA Open ("VISA打开")(error in (no error)=w58, VISA resource name=w57) -> (VISA resource name=w60:refnum<visa-resource-name>, error out=w59:errorcluster)  [unwired: 3 in]
    }
    frame Disabled {
    }
  }
  n4 = Concatenate Strings(w11, "\r\n") -> (w10:string)
  n5 = disable-structure shown="启用" {
    disable-tunnel: w10 -> [w66 _]
    disable-tunnel: w9 -> [w65 w68]
    disable-tunnel: w8 -> [w64 w67]
    disable-tunnel: [w63 w67] -> w7
    disable-tunnel: [w62 w68] -> w5
    frame Disabled {
      n6 = call "RS232_W.vi"("error in (no error)"=w64, "CMD"=w66, "VISA资源名称"=w65) -> ("error out"=w63:errorcluster, "VISA资源名称输出"=w62:refnum<visa-resource-name>)  [unwired: 6 in, 1 out]
    }
    frame Enabled {
    }
  }
  n7 = Concatenate Strings(w14, "\r\n") -> (w19:string)
  n8 = call "Sleep ms.vi"("error in (no error)"=w7, "等待时间（毫秒）"=u32 30) -> ("error out"=w4:errorcluster)  [unwired: 9 in]
  n9 = call "RS232_W.vi"("error in (no error)"=w4, "CMD"=w19, "VISA资源名称"=w5) -> ("error out"=w23:errorcluster, "VISA资源名称输出"=w20:refnum<visa-resource-name>)  [unwired: 6 in, 1 out]
  n10 = Concatenate Strings(w13, "\r\n") -> (w17:string)
  n11 = call "Sleep ms.vi"("error in (no error)"=w23, "等待时间（毫秒）"=u32 200) -> ("error out"=w24:errorcluster)  [unwired: 9 in]
  n12 = call "RS232_W.vi"("error in (no error)"=w24, "CMD"=w17, "VISA资源名称"=w20) -> ("error out"=w21:errorcluster, "VISA资源名称输出"=w16:refnum<visa-resource-name>)  [unwired: 6 in, 1 out]
  n13 = call "Sleep ms.vi"("error in (no error)"=w21, "等待时间（毫秒）"=u32 200) -> ()  [unwired: 9 in, 1 out]
  n14 = VISA Flush I/O Buffer(VISA resource name=w16) -> (VISA resource name out=w39:refnum<visa-resource-name>, error out=w40:errorcluster)  [unwired: 2 in]
  n15 = VISA Write(VISA resource name=w39, write buffer="trig", error in (no error)=w40) -> (VISA resource name out=w34:refnum<visa-resource-name>, error out=w35:errorcluster)  [unwired: 1 out]
  n16 = for {
    N: 2000 -> [_]
    tunnel: w34 -> [w77]
    tunnel: w35 -> [w69]
    tunnel: [w76] -> w37
    tunnel: [w73] -> w36
    stop <- w71 stop-if-true
    n17 = stacked-sequence {
      tunnel: [w79] -> w70
      tunnel: w69 -> [w79]
      frame #0 {
        n18 = Wait (ms)(milliseconds to wait=u32 25 ("等待时间（毫秒）")) -> ()  [unwired: 1 out]
      }
    }
    n19 = property class="Instr"(reference=w77, error in=w70) -> (reference out=w76:refnum<visa-resource-name>, error out=w73:errorcluster, "Bytes at Port"=w75:u32)
    "Serial Settings:Number of Bytes at Serial Port" <- w75
    n20 = Unbundle By Name(w73) -> ("status"=w72:bool)
    n21 = Greater Than 0?(x=w75) -> (x > 0?=w74:bool)
    n22 = Or(x=w72, y=w74) -> (x .or. y?=w71:bool)
  }
  n23 = VISA Read(VISA resource name=w37, byte count=w32, error in (no error)=w36) -> (VISA resource name out=w30:refnum<visa-resource-name>, read buffer=w28:string, return count=w29:u32, error out=w31:errorcluster)
  n24 = case shown="错误" w31 {
    selector: w31 -> [w83 w90]
    tunnel: w30 -> [w82 w89]
    tunnel: [w82 w88] -> w41
    tunnel: [w83 w87] -> w42
    tunnel: [w80 w86] -> w43
    tunnel: [w81 w85] -> w27
    tunnel: w29 -> [w81 w84]
    tunnel: w28 -> [w80 _]
    frame No Error {
    }
    frame Error {
      (unwired) u32 1891 ("字节总数")
      n25 = call <vilib>:"Clear Errors.vi"("error in (no error)"=w90) -> ("error out"=w91:errorcluster)  [unwired: 5 in, 1 out]
      n26 = VISA Write(VISA resource name=w89, write buffer="TRS:DATA?", error in (no error)=w91) -> (VISA resource name out=w93:refnum<visa-resource-name>, error out=w94:errorcluster)  [unwired: 1 out]
      n27 = VISA Read(VISA resource name=w93, byte count=w84, error in (no error)=w94) -> (VISA resource name out=w88:refnum<visa-resource-name>, read buffer=w86:string, return count=w85:u32, error out=w87:errorcluster)
    }
  }
  "read buffer" <- w43
  n28 = Greater Or Equal?(x=w27, y=w32) -> ()  [unwired: 1 out]
  n29 = String Subset(string=w43, length (rest)=w27) -> (substring=w3:string)  [unwired: 1 in]
  "子字符串" <- w3
  n30 = VISA Close(VISA resource name=w41, error in (no error)=w42) -> (error out=w44:errorcluster)
  n31 = for {
    N: 27 -> [_]
    tunnel: w3 -> [w96]
    tunnel: w44 -> [w95]
    tunnel: [w95] -> w1
    i -> [w97]
    n32 = case shown="6" w97 {
      tunnel: w96 -> [w100 w104 w110 w130 w148 w166 w184 w202 w220 w238 w258 w284 w302 w320 w338 w356 w374 w392 w410 w428 w446 w463 w467 w485 w503 w521 w539]
      frame 0, Default {
        n33 = String Subset(string=w100, length (rest)=1 ("长度（剩余）")) -> (substring=→"head":string)  [unwired: 1 in]
      }
      frame 1 {
        n34 = String Subset ("截取字符串")(string=w104, offset (0)=1 ("长度（剩余）"), length (rest)=1 ("长度（剩余）")) -> (substring=→"Primary Sets":string)
      }
      frame 2 {
        n35 = for {
          N: 1600 -> [_]
          shift-right: [w121] -> _
          shift-left: 10 ("长度（剩余）") -> [w118]
          tunnel: w110 -> [w117]
          tunnel: [w113] -> w108 mode=indexing
          tunnel: [w112] -> w105 mode=indexing
          w119 = 4 ("长度（剩余）")
          n36 = Add(x=w119, y=w118) -> (x+y=w121:i32)
          n37 = String Subset(string=w117, offset (0)=w118, length (rest)=w119) -> (substring=w116:string)
          n38 = Reverse String(1:w116) -> (0:w112:string)
          n39 = Type Cast(type=sgl 0.0 ("长度（剩余）"), x=w112) -> (*(type *) &x=w115:sgl)
          n40 = Absolute Value(x=w115) -> (abs(x)=w113:sgl)
          n41 = Multiply(x=w113, y=sgl 1000.0) -> ()  [unwired: 1 out]
        }
        "数组 2" <- w105
        n42 = for {
          N: 40 -> [_]
          shift-right: [w124] -> _
          shift-left: w108 -> [w122]
          tunnel: [w123] -> w106 mode=indexing
          n43 = Split 1D Array(array=w122, index=10 ("索引")) -> (first subarray=w123:sgl[], second subarray=w124:sgl[])
        }
        "Turns Result" <- w106
        n44 = global write "Global.vi" "Turns Result"(w106) -> ()
      }
      frame 3 {
        n45 = for {
          N: 1600 -> [_]
          shift-right: [w139] -> _
          shift-left: 1610 ("长度（剩余）") -> [w135]
          tunnel: w130 -> [w134]
          tunnel: [w132] -> w128 mode=indexing
          w136 = 4 ("长度（剩余）")
          n46 = Add(x=w136, y=w135) -> (x+y=w139:i32)
          n47 = String Subset(string=w134, offset (0)=w135, length (rest)=w136) -> (substring=w133:string)
          n48 = Reverse String(1:w133) -> (0:w138:string)
          n49 = Type Cast(type=sgl 0.0 ("长度（剩余）"), x=w138) -> (*(type *) &x=w132:sgl)
        }
        n50 = for {
          N: 40 -> [_]
          shift-right: [w142] -> _
          shift-left: w128 -> [w140]
          tunnel: [w141] -> w126 mode=indexing
          n51 = Split 1D Array(array=w140, index=10 ("索引")) -> (first subarray=w141:sgl[], second subarray=w142:sgl[])
        }
        "Lx Result" <- w126
        n52 = global write "Global.vi" "Lx Result"(w126) -> ()
      }
      frame 4 {
        n53 = for {
          N: 1600 -> [_]
          shift-right: [w157] -> _
          shift-left: 3210 ("长度（剩余）") -> [w153]
          tunnel: w148 -> [w152]
          tunnel: [w150] -> w146 mode=indexing
          w154 = 4 ("长度（剩余）")
          n54 = Add(x=w154, y=w153) -> (x+y=w157:i32)
          n55 = String Subset(string=w152, offset (0)=w153, length (rest)=w154) -> (substring=w151:string)
          n56 = Reverse String(1:w151) -> (0:w156:string)
          n57 = Type Cast(type=sgl 0.0 ("长度（剩余）"), x=w156) -> (*(type *) &x=w150:sgl)
        }
        n58 = for {
          N: 40 -> [_]
          shift-right: [w160] -> _
          shift-left: w146 -> [w158]
          tunnel: [w159] -> w144 mode=indexing
          n59 = Split 1D Array(array=w158, index=10 ("索引")) -> (first subarray=w159:sgl[], second subarray=w160:sgl[])
        }
        "Lk Result" <- w144
        n60 = global write "Global.vi" "Lk Result"(w144) -> ()
      }
      frame 5 {
        n61 = for {
          N: 40 -> [_]
          shift-right: [w175] -> _
          shift-left: 490 ("长度（剩余）") -> [w171]
          tunnel: w166 -> [w170]
          tunnel: [w168] -> w164 mode=indexing
          w172 = 4 ("长度（剩余）")
          n62 = Add(x=w172, y=w171) -> (x+y=w175:i32)
          n63 = String Subset(string=w170, offset (0)=w171, length (rest)=w172) -> (substring=w169:string)
          n64 = Reverse String(1:w169) -> (0:w174:string)
          n65 = Type Cast(type=sgl 0.0 ("长度（剩余）"), x=w174) -> (*(type *) &x=w168:sgl)
        }
        n66 = for {
          N: 4 -> [_]
          shift-right: [w178] -> _
          shift-left: w164 -> [w176]
          tunnel: [w177] -> w162 mode=indexing
          n67 = Split 1D Array(array=w176, index=10 ("索引")) -> (first subarray=w177:sgl[], second subarray=w178:sgl[])
        }
        "Cx Result" <- w162
      }
      frame 6 {
        n68 = for {
          N: 1600 -> [_]
          shift-right: [w193] -> _
          shift-left: 6410 ("长度（剩余）") -> [w189]
          tunnel: w184 -> [w188]
          tunnel: [w186] -> w182 mode=indexing
          w190 = 4 ("长度（剩余）")
          n69 = Add(x=w190, y=w189) -> (x+y=w193:i32)
          n70 = String Subset "截取字符串"(string=w188, offset (0)=w189, length (rest)=w190) -> (substring=w187:string)
          n71 = Reverse String "反转字符串"(1:w187) -> (0:w192:string)
          n72 = Type Cast(type=sgl 0.0 ("长度（剩余）"), x=w192) -> (*(type *) &x=w186:sgl)
        }
        "数组" <- w182
        n73 = for {
          N: 40 -> [_]
          shift-right: [w196] -> _
          shift-left: w182 -> [w194]
          tunnel: [w195] -> w180 mode=indexing
          n74 = Split 1D Array "拆分一维数组"(array=w194, index=10 ("索引")) -> (first subarray=w195:sgl[], second subarray=w196:sgl[])
        }
        "DCR Result" <- w180
        n75 = global write "Global.vi" "DCR Result"(w180) -> ()
      }
      frame 7 {
        n76 = for {
          N: 40 -> [_]
          shift-right: [w211] -> _
          shift-left: 810 ("长度（剩余）") -> [w207]
          tunnel: w202 -> [w206]
          tunnel: [w204] -> w200 mode=indexing
          w208 = 4 ("长度（剩余）")
          n77 = Add(x=w208, y=w207) -> (x+y=w211:i32)
          n78 = String Subset(string=w206, offset (0)=w207, length (rest)=w208) -> (substring=w205:string)
          n79 = Reverse String(1:w205) -> (0:w210:string)
          n80 = Type Cast(type=sgl 0.0 ("长度（剩余）"), x=w210) -> (*(type *) &x=w204:sgl)
        }
        n81 = for {
          N: 4 -> [_]
          shift-right: [w214] -> _
          shift-left: w200 -> [w212]
          tunnel: [w213] -> w198 mode=indexing
          n82 = Split 1D Array(array=w212, index=10 ("索引")) -> (first subarray=w213:sgl[], second subarray=w214:sgl[])
        }
        "LxQ Result" <- w198
      }
      frame 8 {
        n83 = for {
          N: 40 -> [_]
          shift-right: [w229] -> _
          shift-left: 970 ("长度（剩余）") -> [w225]
          tunnel: w220 -> [w224]
          tunnel: [w222] -> w218 mode=indexing
          w226 = 4 ("长度（剩余）")
          n84 = Add(x=w226, y=w225) -> (x+y=w229:i32)
          n85 = String Subset(string=w224, offset (0)=w225, length (rest)=w226) -> (substring=w223:string)
          n86 = Reverse String(1:w223) -> (0:w228:string)
          n87 = Type Cast(type=sgl 0.0 ("长度（剩余）"), x=w228) -> (*(type *) &x=w222:sgl)
        }
        n88 = for {
          N: 4 -> [_]
          shift-right: [w232] -> _
          shift-left: w218 -> [w230]
          tunnel: [w231] -> w216 mode=indexing
          n89 = Split 1D Array(array=w230, index=10 ("索引")) -> (first subarray=w231:sgl[], second subarray=w232:sgl[])
        }
        "ACR Result" <- w216
      }
      frame 9 {
        n90 = for {
          N: 40 -> [_]
          shift-right: [w247] -> _
          shift-left: 1130 ("长度（剩余）") -> [w243]
          tunnel: w238 -> [w242]
          tunnel: [w240] -> w236 mode=indexing
          w244 = 4 ("长度（剩余）")
          n91 = Add(x=w244, y=w243) -> (x+y=w247:i32)
          n92 = String Subset(string=w242, offset (0)=w243, length (rest)=w244) -> (substring=w241:string)
          n93 = Reverse String(1:w241) -> (0:w246:string)
          n94 = Type Cast(type=sgl 0.0 ("长度（剩余）"), x=w246) -> (*(type *) &x=w240:sgl)
        }
        n95 = for {
          N: 4 -> [_]
          shift-right: [w250] -> _
          shift-left: w236 -> [w248]
          tunnel: [w249] -> w234 mode=indexing
          n96 = Split 1D Array(array=w248, index=10 ("索引")) -> (first subarray=w249:sgl[], second subarray=w250:sgl[])
        }
        "Zx Result" <- w234
      }
      frame 10 {
        (unwired) 1290 ("长度（剩余）")
        (unwired) 4
        n97 = for {
          N: 400 -> [_]
          shift-right: [w275] -> _
          shift-left: 12810 ("长度（剩余）") -> [w272]
          tunnel: w258 -> [w271]
          tunnel: [w269] -> w253 mode=indexing
          w273 = 1 ("长度（剩余）")
          n98 = Add(x=w273, y=w272) -> (x+y=w275:i32)
          n99 = String Subset(string=w271, offset (0)=w272, length (rest)=w273) -> (substring=w270:string)
          n100 = Reverse String(1:w270) -> (0:w274:string)
          n101 = Type Cast(type="", x=w274) -> (*(type *) &x=w269:string)
        }
        n102 = for {
          N: 40 -> [_]
          shift-right: [w278] -> _
          shift-left: w253 -> [w276]
          tunnel: [w277] -> w252 mode=indexing
          n103 = Split 1D Array(array=w276, index=10 ("索引")) -> (first subarray=w277:string[], second subarray=w278:string[])
        }
        "Polarity Result1" <- w252
        n104 = for {
          N: 40 -> [_]
          tunnel: w252 -> [w261] mode=indexing
          tunnel: [w260] -> w254 mode=indexing
          n105 = for {
            N: 10 -> [_]
            tunnel: w261 -> [w264] mode=indexing
            tunnel: [w263] -> w260 mode=indexing
            n106 = case shown="\" \", 默认" w264 {
              tunnel: [u8 4 u8 1 u8 0] -> w263
              frame "-" {
              }
              frame "+" {
              }
              frame " ", Default {
              }
            }
          }
        }
        "Polarity Result" <- w254
      }
      frame 11 {
        n107 = for {
          N: 40 -> [_]
          shift-right: [w293] -> _
          shift-left: 1330 ("长度（剩余）") -> [w289]
          tunnel: w284 -> [w288]
          tunnel: [w286] -> w282 mode=indexing
          w290 = 1 ("长度（剩余）")
          n108 = Add(x=w290, y=w289) -> (x+y=w293:i32)
          n109 = String Subset ("截取字符串")(string=w288, offset (0)=w289, length (rest)=w290) -> (substring=w287:string)
          n110 = Reverse String(1:w287) -> (0:w292:string)
          n111 = Type Cast(type=u8 0 ("长度（剩余）"), x=w292) -> (*(type *) &x=w286:u8)
        }
        n112 = for {
          N: 4 -> [_]
          shift-right: [w296] -> _
          shift-left: w282 -> [w294]
          tunnel: [w295] -> w280 mode=indexing
          n113 = Split 1D Array(array=w294, index=10 ("索引")) -> (first subarray=w295:u8[], second subarray=w296:u8[])
        }
        "Turns Compare Result" <- w280
      }
      frame 12 {
        n114 = for {
          N: 40 -> [_]
          shift-right: [w311] -> _
          shift-left: 1370 ("长度（剩余）") -> [w307]
          tunnel: w302 -> [w306]
          tunnel: [w304] -> w300 mode=indexing
          w308 = 1 ("长度（剩余）")
          n115 = Add(x=w308, y=w307) -> (x+y=w311:i32)
          n116 = String Subset(string=w306, offset (0)=w307, length (rest)=w308) -> (substring=w305:string)
          n117 = Reverse String(1:w305) -> (0:w310:string)
          n118 = Type Cast(type=u8 0 ("长度（剩余）"), x=w310) -> (*(type *) &x=w304:u8)
        }
        n119 = for {
          N: 4 -> [_]
          shift-right: [w314] -> _
          shift-left: w300 -> [w312]
          tunnel: [w313] -> w298 mode=indexing
          n120 = Split 1D Array(array=w312, index=10 ("索引")) -> (first subarray=w313:u8[], second subarray=w314:u8[])
        }
        "Lx Compare Result" <- w298
      }
      frame 13 {
        n121 = for {
          N: 40 -> [_]
          shift-right: [w329] -> _
          shift-left: 1410 ("长度（剩余）") -> [w325]
          tunnel: w320 -> [w324]
          tunnel: [w322] -> w318 mode=indexing
          w326 = 1 ("长度（剩余）")
          n122 = Add(x=w326, y=w325) -> (x+y=w329:i32)
          n123 = String Subset(string=w324, offset (0)=w325, length (rest)=w326) -> (substring=w323:string)
          n124 = Reverse String(1:w323) -> (0:w328:string)
          n125 = Type Cast(type=u8 0 ("长度（剩余）"), x=w328) -> (*(type *) &x=w322:u8)
        }
        n126 = for {
          N: 4 -> [_]
          shift-right: [w332] -> _
          shift-left: w318 -> [w330]
          tunnel: [w331] -> w316 mode=indexing
          n127 = Split 1D Array(array=w330, index=10 ("索引")) -> (first subarray=w331:u8[], second subarray=w332:u8[])
        }
        "Lk Compare Result" <- w316
      }
      frame 14 {
        n128 = for {
          N: 40 -> [_]
          shift-right: [w347] -> _
          shift-left: 1450 ("长度（剩余）") -> [w343]
          tunnel: w338 -> [w342]
          tunnel: [w340] -> w336 mode=indexing
          w344 = 1 ("长度（剩余）")
          n129 = Add(x=w344, y=w343) -> (x+y=w347:i32)
          n130 = String Subset(string=w342, offset (0)=w343, length (rest)=w344) -> (substring=w341:string)
          n131 = Reverse String(1:w341) -> (0:w346:string)
          n132 = Type Cast(type=u8 0 ("长度（剩余）"), x=w346) -> (*(type *) &x=w340:u8)
        }
        n133 = for {
          N: 4 -> [_]
          shift-right: [w350] -> _
          shift-left: w336 -> [w348]
          tunnel: [w349] -> w334 mode=indexing
          n134 = Split 1D Array(array=w348, index=10 ("索引")) -> (first subarray=w349:u8[], second subarray=w350:u8[])
        }
        "C Compare Result" <- w334
      }
      frame 15 {
        n135 = for {
          N: 40 -> [_]
          shift-right: [w365] -> _
          shift-left: 1490 ("长度（剩余）") -> [w361]
          tunnel: w356 -> [w360]
          tunnel: [w358] -> w354 mode=indexing
          w362 = 1 ("长度（剩余）")
          n136 = Add(x=w362, y=w361) -> (x+y=w365:i32)
          n137 = String Subset(string=w360, offset (0)=w361, length (rest)=w362) -> (substring=w359:string)
          n138 = Reverse String(1:w359) -> (0:w364:string)
          n139 = Type Cast(type=u8 0 ("长度（剩余）"), x=w364) -> (*(type *) &x=w358:u8)
        }
        n140 = for {
          N: 4 -> [_]
          shift-right: [w368] -> _
          shift-left: w354 -> [w366]
          tunnel: [w367] -> w352 mode=indexing
          n141 = Split 1D Array(array=w366, index=10 ("索引")) -> (first subarray=w367:u8[], second subarray=w368:u8[])
        }
        "DCR Compare Result" <- w352
      }
      frame 16 {
        n142 = for {
          N: 40 -> [_]
          shift-right: [w383] -> _
          shift-left: 1530 ("长度（剩余）") -> [w379]
          tunnel: w374 -> [w378]
          tunnel: [w376] -> w372 mode=indexing
          w380 = 1 ("长度（剩余）")
          n143 = Add(x=w380, y=w379) -> (x+y=w383:i32)
          n144 = String Subset(string=w378, offset (0)=w379, length (rest)=w380) -> (substring=w377:string)
          n145 = Reverse String(1:w377) -> (0:w382:string)
          n146 = Type Cast(type=u8 0 ("长度（剩余）"), x=w382) -> (*(type *) &x=w376:u8)
        }
        n147 = for {
          N: 4 -> [_]
          shift-right: [w386] -> _
          shift-left: w372 -> [w384]
          tunnel: [w385] -> w370 mode=indexing
          n148 = Split 1D Array(array=w384, index=10 ("索引")) -> (first subarray=w385:u8[], second subarray=w386:u8[])
        }
        "LxQ Compare Result" <- w370
      }
      frame 17 {
        n149 = for {
          N: 40 -> [_]
          shift-right: [w401] -> _
          shift-left: 1570 ("长度（剩余）") -> [w395]
          tunnel: w392 -> [w396]
          tunnel: [w397] -> w390 mode=indexing
          w394 = 1 ("长度（剩余）")
          n150 = Add(x=w394, y=w395) -> (x+y=w401:i32)
          n151 = String Subset(string=w396, offset (0)=w395, length (rest)=w394) -> (substring=w398:string)
          n152 = Reverse String(1:w398) -> (0:w400:string)
          n153 = Type Cast(type=u8 0 ("长度（剩余）"), x=w400) -> (*(type *) &x=w397:u8)
        }
        n154 = for {
          N: 4 -> [_]
          shift-right: [w404] -> _
          shift-left: w390 -> [w402]
          tunnel: [w403] -> w388 mode=indexing
          n155 = Split 1D Array(array=w402, index=10 ("索引")) -> (first subarray=w403:u8[], second subarray=w404:u8[])
        }
        "Rs Compare Result" <- w388
      }
      frame 18 {
        n156 = for {
          N: 40 -> [_]
          shift-right: [w419] -> _
          shift-left: 1610 ("长度（剩余）") -> [w413]
          tunnel: w410 -> [w414]
          tunnel: [w415] -> w408 mode=indexing
          w412 = 1 ("长度（剩余）")
          n157 = Add(x=w412, y=w413) -> (x+y=w419:i32)
          n158 = String Subset(string=w414, offset (0)=w413, length (rest)=w412) -> (substring=w416:string)
          n159 = Reverse String(1:w416) -> (0:w418:string)
          n160 = Type Cast(type=u8 0 ("长度（剩余）"), x=w418) -> (*(type *) &x=w415:u8)
        }
        n161 = for {
          N: 4 -> [_]
          shift-right: [w422] -> _
          shift-left: w408 -> [w420]
          tunnel: [w421] -> w406 mode=indexing
          n162 = Split 1D Array(array=w420, index=10 ("索引")) -> (first subarray=w421:u8[], second subarray=w422:u8[])
        }
        "Z Compare Result" <- w406
      }
      frame 19 {
        n163 = for {
          N: 40 -> [_]
          shift-right: [w437] -> _
          shift-left: 1650 ("长度（剩余）") -> [w432]
          tunnel: w428 -> [w433]
          tunnel: [w434] -> w426 mode=indexing
          w431 = 1 ("长度（剩余）")
          n164 = Add(x=w431, y=w432) -> (x+y=w437:i32)
          n165 = String Subset(string=w433, offset (0)=w432, length (rest)=w431) -> (substring=w435:string)
          n166 = Reverse String(1:w435) -> (0:w436:string)
          n167 = Type Cast(type=u8 0 ("长度（剩余）"), x=w436) -> (*(type *) &x=w434:u8)
        }
        n168 = for {
          N: 4 -> [_]
          shift-right: [w440] -> _
          shift-left: w426 -> [w438]
          tunnel: [w439] -> w424 mode=indexing
          n169 = Split 1D Array(array=w438, index=10 ("索引")) -> (first subarray=w439:u8[], second subarray=w440:u8[])
        }
        "Balance Compare Result" <- w424
      }
      frame 20 {
        n170 = for {
          N: 40 -> [_]
          shift-right: [w455] -> _
          shift-left: 1690 ("长度（剩余）") -> [w450]
          tunnel: w446 -> [w451]
          tunnel: [w452] -> w444 mode=indexing
          w449 = 1 ("长度（剩余）")
          n171 = Add(x=w449, y=w450) -> (x+y=w455:i32)
          n172 = String Subset(string=w451, offset (0)=w450, length (rest)=w449) -> (substring=w453:string)
          n173 = Reverse String(1:w453) -> (0:w454:string)
          n174 = Type Cast(type=u8 0 ("长度（剩余）"), x=w454) -> (*(type *) &x=w452:u8)
        }
        n175 = for {
          N: 4 -> [_]
          shift-right: [w458] -> _
          shift-left: w444 -> [w456]
          tunnel: [w457] -> w442 mode=indexing
          n176 = Split 1D Array(array=w456, index=10 ("索引")) -> (first subarray=w457:u8[], second subarray=w458:u8[])
        }
        "PS Compare Result" <- w442
      }
      frame 21 {
        n177 = String Subset(string=w463, offset (0)=1730 ("长度（剩余）"), length (rest)=1 ("长度（剩余）")) -> (substring=w466:string)
        n178 = Reverse String(1:w466) -> (0:w464:string)
        n179 = Type Cast(type=u8 0 ("长度（剩余）"), x=w464) -> (*(type *) &x=→"总判断":u8)
      }
      frame 22 {
        n180 = for {
          N: 20 -> [_]
          shift-right: [w480] -> _
          shift-left: 1731 ("长度（剩余）") -> [w476]
          tunnel: w467 -> [w475]
          tunnel: [w473] -> w470 mode=indexing
          w477 = 4 ("长度（剩余）")
          n181 = Add(x=w477, y=w476) -> (x+y=w480:i32)
          n182 = String Subset(string=w475, offset (0)=w476, length (rest)=w477) -> (substring=w474:string)
          n183 = Reverse String(1:w474) -> (0:w479:string)
          n184 = Type Cast(type=sgl 0.0 ("长度（剩余）"), x=w479) -> (*(type *) &x=w473:sgl)
        }
        n185 = for {
          N: 4 -> [_]
          shift-right: [w483] -> _
          shift-left: w470 -> [w481]
          tunnel: [w482] -> w468 mode=indexing
          n186 = Split 1D Array(array=w481, index=5 ("索引")) -> (first subarray=w482:sgl[], second subarray=w483:sgl[])
        }
        "Bls Result" <- w468
      }
      frame 23 {
        n187 = for {
          N: 8 -> [_]
          shift-right: [w498] -> _
          shift-left: 1811 ("长度（剩余）") -> [w494]
          tunnel: w485 -> [w493]
          tunnel: [w491] -> w487 mode=indexing
          w495 = 4 ("长度（剩余）")
          n188 = Add(x=w495, y=w494) -> (x+y=w498:i32)
          n189 = String Subset(string=w493, offset (0)=w494, length (rest)=w495) -> (substring=w492:string)
          n190 = Reverse String(1:w492) -> (0:w497:string)
          n191 = Type Cast(type=sgl 0.0 ("长度（剩余）"), x=w497) -> (*(type *) &x=w491:sgl)
        }
        n192 = for {
          N: 4 -> [_]
          shift-right: [w501] -> _
          shift-left: w487 -> [w499]
          tunnel: [w500] -> w490 mode=indexing
          n193 = Split 1D Array(array=w499, index=2 ("索引")) -> (first subarray=w500:sgl[], second subarray=w501:sgl[])
        }
        "LED VfResult" <- w490
      }
      frame 24 {
        n194 = for {
          N: 8 -> [_]
          shift-right: [w516] -> _
          shift-left: 1843 ("长度（剩余）") -> [w512]
          tunnel: w503 -> [w511]
          tunnel: [w509] -> w505 mode=indexing
          w513 = 4 ("长度（剩余）")
          n195 = Add(x=w513, y=w512) -> (x+y=w516:i32)
          n196 = String Subset(string=w511, offset (0)=w512, length (rest)=w513) -> (substring=w510:string)
          n197 = Reverse String(1:w510) -> (0:w515:string)
          n198 = Type Cast(type=sgl 0.0 ("长度（剩余）"), x=w515) -> (*(type *) &x=w509:sgl)
        }
        n199 = for {
          N: 4 -> [_]
          shift-right: [w519] -> _
          shift-left: w505 -> [w517]
          tunnel: [w518] -> w508 mode=indexing
          n200 = Split 1D Array(array=w517, index=2 ("索引")) -> (first subarray=w518:sgl[], second subarray=w519:sgl[])
        }
        "LED IrResult" <- w508
      }
      frame 25 {
        n201 = for {
          N: 8 -> [_]
          shift-right: [w534] -> _
          shift-left: 1875 ("长度（剩余）") -> [w529]
          tunnel: w521 -> [w530]
          tunnel: [w531] -> w523 mode=indexing
          w528 = 1 ("长度（剩余）")
          n202 = Add(x=w528, y=w529) -> (x+y=w534:i32)
          n203 = String Subset(string=w530, offset (0)=w529, length (rest)=w528) -> (substring=w532:string)
          n204 = Reverse String(1:w532) -> (0:w533:string)
          n205 = Type Cast(type=u8 0 ("长度（剩余）"), x=w533) -> (*(type *) &x=w531:u8)
        }
        n206 = for {
          N: 4 -> [_]
          shift-right: [w537] -> _
          shift-left: w523 -> [w535]
          tunnel: [w536] -> w526 mode=indexing
          n207 = Split 1D Array(array=w535, index=2 ("索引")) -> (first subarray=w536:u8[], second subarray=w537:u8[])
        }
        "LED VfCompare Result" <- w526
      }
      frame 26 {
        n208 = for {
          N: 8 -> [_]
          shift-right: [w552] -> _
          shift-left: 1883 ("长度（剩余）") -> [w547]
          tunnel: w539 -> [w548]
          tunnel: [w549] -> w541 mode=indexing
          w546 = 1 ("长度（剩余）")
          n209 = Add(x=w546, y=w547) -> (x+y=w552:i32)
          n210 = String Subset(string=w548, offset (0)=w547, length (rest)=w546) -> (substring=w550:string)
          n211 = Reverse String(1:w550) -> (0:w551:string)
          n212 = Type Cast(type=u8 0 ("长度（剩余）"), x=w551) -> (*(type *) &x=w549:u8)
        }
        n213 = for {
          N: 4 -> [_]
          shift-right: [w555] -> _
          shift-left: w541 -> [w553]
          tunnel: [w554] -> w544 mode=indexing
          n214 = Split 1D Array(array=w553, index=2 ("索引")) -> (first subarray=w554:u8[], second subarray=w555:u8[])
        }
        "LED IrCompare Result" <- w544
      }
    }
  }
  "error out" <- w1
